vi "Main.vi"() -> ()   [LabVIEW 2020]
uses:
  Action control.ctl
  Script control.ctl
  Joystick controls.ctl
  <vilib>/Platform/TimedLoop/XDataNode/timing_clust.ctl
  <vilib>/Platform/TimedLoop/XDataNode/nitl_modes.ctl
  <vilib>/Platform/TimedLoop/XDataNode/wakeup.ctl
  8df4f0e3-bdc8-4595-ad00-b98df174246d.vi
  <vilib>/High Genius/HG_WSI_Tookit/Dependencies/Library/IMU/IMU.lvclass
  C:/Program Files (x86)/National Instruments/LabVIEW 2020/vi.lib/High Genius/HG_WSI_Tookit/Dependencies/Library/HG_LIB/HG_LIB.lvclass
  <vilib>/High Genius/HG_WSI_Tookit/Dependencies/Library/Analog In/Analog In.lvclass
  <vilib>/High Genius/HG_WSI_Tookit/Dependencies/Library/PWM/PWM.lvclass
  <vilib>/High Genius/HG_WSI_Tookit/Dependencies/Library/Digital Input and Output/Digital Input and Output.lvclass
  <vilib>/High Genius/HG_WSI_Tookit/Dependencies/Library/TitanENC/TitanENC.lvclass
  <vilib>/High Genius/HG_WSI_Tookit/Dependencies/Library/CAN/CAN.lvclass
  <vilib>/High Genius/HG_WSI_Tookit/Dependencies/Library/IIC/IIC.lvclass
  <vilib>/High Genius/HG_WSI_Tookit/Dependencies/Library/ISQ/ISQ.lvclass
  <vilib>/High Genius/HG_WSI_Tookit/Dependencies/Library/Pulse/Pulse.lvclass
  <vilib>/Platform/TimedLoop/XDataNode/XDataNode.xnode
  <vilib>/High Genius/HG_WSI_Tookit/Dependencies/Library/HG_LIB/HG_LIB.lvclass
  <vilib>/Platform/TimedLoop/XDataNode/XDNodeRunTimeDep.lvlib
panel:
  out "Waveform Chart 2":dbl(graph)=40.0
  out "Waveform Chart":dbl(graph)
  out "Volage":dbl(knob) scale=12.0..15.0
  in  "GPS Start":cluster{"X":dbl, "Y":dbl, "Angle ":i16}={"X"=166.0, "Y"=34.0, "Angle "=90}
  in  "GPS True":cluster{"X":dbl, "Y":dbl, "Z":dbl}
  in  "GPS":cluster{"X":dbl, "Y":dbl, "Angle ":i16}
  in  "Set GPS":cluster{"Set":bool, "X":dbl, "Y":dbl, "Z":dbl}
  in  "Block Rotate":bool
  in  "Tab Script":T1(tab)
  out "Array 0":T3(array[cluster])=[{"Activ"=FALSE, "X"=0.0, "Y"=0.0, "Z"=0.0, "Div"=0, "Set 1"=FALSE, "Set 2"=FALSE, "Set 3"=FALSE, "Skip"=FALSE, "action"=enum."Start"}, {"Activ"=FALSE, "X"=200.0, "Y"=113.0, "Z"=0.0, "Div"=0, "Set 1"=FALSE, "Set 2"=FALSE, "Set 3"=FALSE, "Skip"=FALSE, "action"=enum."Move"}, {"Activ"=FALSE, "X"=3.0, "Y"=0.0, "Z"=0.0, "Div"=0, "Set 1"=FALSE, "Set 2"=FALSE, "Set 3"=FALSE, "Skip"=FALSE, "action"=enum."Smooth pause"}, {"Activ"=FALSE, "X"=0.0, "Y"=0.0, "Z"=0.0, "Div"=0, "Set 1"=FALSE, "Set 2"=FALSE, "Set 3"=FALSE, "Skip"=FALSE, "action"=enum."Move"}, {"Activ"=FALSE, "X"=200.0, "Y"=50.0, "Z"=0.0, "Div"=0, "Set 1"=FALSE, "Set 2"=FALSE, "Set 3"=FALSE, "Skip"=FALSE, "action"=enum."Move"}, {"Activ"=FALSE, "X"=1.0, "Y"=0.0, "Z"=0.0, "Div"=0, "Set 1"=FALSE, "Set 2"=FALSE, "Set 3"=FALSE, "Skip"=FALSE, "action"=enum."Smooth pause"}, {"Activ"=FALSE, "X"=90.0, "Y"=0.0, "Z"=0.0, "Div"=0, "Set 1"=FALSE, "Set 2"=FALSE, "Set 3"=FALSE, "Skip"=FALSE, "action"=enum."Rotation"}, {"Activ"=FALSE, "X"=90.0, "Y"=0.0, "Z"=0.0, "Div"=0, "Set 1"=FALSE, "Set 2"=FALSE, "Set 3"=FALSE, "Skip"=FALSE, "action"=enum."Rotation"}, {"Activ"=FALSE, "X"=90.0, "Y"=0.0, "Z"=0.0, "Div"=0, "Set 1"=FALSE, "Set 2"=FALSE, "Set 3"=FALSE, "Skip"=FALSE, "action"=enum."Rotation"}, {"Activ"=FALSE, "X"=1.0, "Y"=0.0, "Z"=0.0, "Div"=0, "Set 1"=FALSE, "Set 2"=FALSE, "Set 3"=FALSE, "Skip"=FALSE, "action"=enum."Smooth pause"}, {"Activ"=FALSE, "X"=90.0, "Y"=0.0, "Z"=0.0, "Div"=0, "Set 1"=FALSE, "Set 2"=FALSE, "Set 3"=FALSE, "Skip"=FALSE, "action"=enum."Rotation Correct"}, {"Activ"=TRUE, "X"=0.0, "Y"=0.0, "Z"=0.0, "Div"=0, "Set 1"=FALSE, "Set 2"=FALSE, "Set 3"=FALSE, "Skip"=FALSE, "action"=enum."End"}]
  in  "Array 1":T3(array[cluster])=[{"Activ"=FALSE, "X"=0.0, "Y"=0.0, "Z"=0.0, "Div"=0, "Set 1"=FALSE, "Set 2"=FALSE, "Set 3"=FALSE, "Skip"=FALSE, "action"=enum."Start"}, {"Activ"=FALSE, "X"=0.0, "Y"=0.0, "Z"=0.0, "Div"=0, "Set 1"=FALSE, "Set 2"=FALSE, "Set 3"=FALSE, "Skip"=FALSE, "action"=enum."Gamepad"}, {"Activ"=FALSE, "X"=0.0, "Y"=0.0, "Z"=0.0, "Div"=0, "Set 1"=FALSE, "Set 2"=FALSE, "Set 3"=FALSE, "Skip"=FALSE, "action"=enum."Pause"}, {"Activ"=FALSE, "X"=0.0, "Y"=0.0, "Z"=0.0, "Div"=0, "Set 1"=FALSE, "Set 2"=FALSE, "Set 3"=FALSE, "Skip"=FALSE, "action"=enum."End"}]
  in  "Array 2":T3(array[cluster])=[{"Activ"=FALSE, "X"=0.0, "Y"=0.0, "Z"=0.0, "Div"=0, "Set 1"=FALSE, "Set 2"=FALSE, "Set 3"=FALSE, "Skip"=FALSE, "action"=enum."Start"}, {"Activ"=FALSE, "X"=200.0, "Y"=45.0, "Z"=0.0, "Div"=0, "Set 1"=FALSE, "Set 2"=FALSE, "Set 3"=FALSE, "Skip"=FALSE, "action"=enum."Move"}, {"Activ"=FALSE, "X"=1.0, "Y"=0.0, "Z"=0.0, "Div"=0, "Set 1"=FALSE, "Set 2"=FALSE, "Set 3"=FALSE, "Skip"=FALSE, "action"=enum."Smooth pause"}, {"Activ"=FALSE, "X"=0.0, "Y"=0.0, "Z"=0.0, "Div"=0, "Set 1"=FALSE, "Set 2"=FALSE, "Set 3"=FALSE, "Skip"=FALSE, "action"=enum."End"}]
  in  "Array 3":T3(array[cluster])=[{"Activ"=FALSE, "X"=0.0, "Y"=0.0, "Z"=0.0, "Div"=0, "Set 1"=FALSE, "Set 2"=FALSE, "Set 3"=FALSE, "Skip"=FALSE, "action"=enum."Start"}, {"Activ"=FALSE, "X"=90.0, "Y"=0.0, "Z"=0.0, "Div"=0, "Set 1"=FALSE, "Set 2"=FALSE, "Set 3"=FALSE, "Skip"=FALSE, "action"=enum."Rotation"}, {"Activ"=FALSE, "X"=90.0, "Y"=0.0, "Z"=0.0, "Div"=0, "Set 1"=FALSE, "Set 2"=FALSE, "Set 3"=FALSE, "Skip"=FALSE, "action"=enum."Rotation"}, {"Activ"=FALSE, "X"=1.0, "Y"=0.0, "Z"=0.0, "Div"=0, "Set 1"=FALSE, "Set 2"=FALSE, "Set 3"=FALSE, "Skip"=FALSE, "action"=enum."Smooth pause"}, {"Activ"=FALSE, "X"=90.0, "Y"=0.0, "Z"=0.0, "Div"=0, "Set 1"=FALSE, "Set 2"=FALSE, "Set 3"=FALSE, "Skip"=FALSE, "action"=enum."Rotation Correct"}, {"Activ"=FALSE, "X"=1.0, "Y"=0.0, "Z"=0.0, "Div"=0, "Set 1"=FALSE, "Set 2"=FALSE, "Set 3"=FALSE, "Skip"=FALSE, "action"=enum."Smooth pause"}, {"Activ"=FALSE, "X"=70.0, "Y"=0.0, "Z"=0.0, "Div"=0, "Set 1"=FALSE, "Set 2"=FALSE, "Set 3"=FALSE, "Skip"=FALSE, "action"=enum."Move"}, {"Activ"=FALSE, "X"=1.0, "Y"=0.0, "Z"=0.0, "Div"=0, "Set 1"=FALSE, "Set 2"=FALSE, "Set 3"=FALSE, "Skip"=FALSE, "action"=enum."Smooth pause"}, {"Activ"=FALSE, "X"=180.0, "Y"=0.0, "Z"=0.0, "Div"=0, "Set 1"=FALSE, "Set 2"=FALSE, "Set 3"=FALSE, "Skip"=FALSE, "action"=enum."Rotation"}, {"Activ"=FALSE, "X"=90.0, "Y"=0.0, "Z"=0.0, "Div"=0, "Set 1"=FALSE, "Set 2"=FALSE, "Set 3"=FALSE, "Skip"=FALSE, "action"=enum."Rotation"}, {"Activ"=FALSE, "X"=1.0, "Y"=0.0, "Z"=0.0, "Div"=0, "Set 1"=FALSE, "Set 2"=FALSE, "Set 3"=FALSE, "Skip"=FALSE, "action"=enum."Smooth pause"}, {"Activ"=FALSE, "X"=90.0, "Y"=0.0, "Z"=0.0, "Div"=0, "Set 1"=FALSE, "Set 2"=FALSE, "Set 3"=FALSE, "Skip"=FALSE, "action"=enum."Rotation Correct"}, {"Activ"=FALSE, "X"=1.0, "Y"=0.0, "Z"=0.0, "Div"=0, "Set 1"=FALSE, "Set 2"=FALSE, "Set 3"=FALSE, "Skip"=FALSE, "action"=enum."Smooth pause"}, {"Activ"=FALSE, "X"=240.0, "Y"=40.0, "Z"=0.0, "Div"=0, "Set 1"=FALSE, "Set 2"=FALSE, "Set 3"=FALSE, "Skip"=FALSE, "action"=enum."Move"}, {"Activ"=FALSE, "X"=1.0, "Y"=0.0, "Z"=0.0, "Div"=0, "Set 1"=FALSE, "Set 2"=FALSE, "Set 3"=FALSE, "Skip"=FALSE, "action"=enum."Smooth pause"}, {"Activ"=FALSE, "X"=-90.0, "Y"=0.0, "Z"=0.0, "Div"=0, "Set 1"=FALSE, "Set 2"=FALSE, "Set 3"=FALSE, "Skip"=FALSE, "action"=enum."Rotation"}, {"Activ"=FALSE, "X"=1.0, "Y"=0.0, "Z"=0.0, "Div"=0, "Set 1"=FALSE, "Set 2"=FALSE, "Set 3"=FALSE, "Skip"=FALSE, "action"=enum."Smooth pause"}, {"Activ"=FALSE, "X"=1.0, "Y"=0.0, "Z"=0.0, "Div"=0, "Set 1"=FALSE, "Set 2"=FALSE, "Set 3"=FALSE, "Skip"=FALSE, "action"=enum."Smooth pause"}, {"Activ"=FALSE, "X"=50.0, "Y"=0.0, "Z"=0.0, "Div"=0, "Set 1"=FALSE, "Set 2"=FALSE, "Set 3"=FALSE, "Skip"=FALSE, "action"=enum."Move"}, {"Activ"=FALSE, "X"=1.0, "Y"=0.0, "Z"=0.0, "Div"=0, "Set 1"=FALSE, "Set 2"=FALSE, "Set 3"=FALSE, "Skip"=FALSE, "action"=enum."Smooth pause"}, {"Activ"=FALSE, "X"=720.0, "Y"=0.0, "Z"=0.0, "Div"=0, "Set 1"=FALSE, "Set 2"=FALSE, "Set 3"=FALSE, "Skip"=FALSE, "action"=enum."Rotation"}, {"Activ"=FALSE, "X"=1.0, "Y"=0.0, "Z"=0.0, "Div"=0, "Set 1"=FALSE, "Set 2"=FALSE, "Set 3"=FALSE, "Skip"=FALSE, "action"=enum."Smooth pause"}, {"Activ"=FALSE, "X"=0.0, "Y"=0.0, "Z"=0.0, "Div"=0, "Set 1"=FALSE, "Set 2"=FALSE, "Set 3"=FALSE, "Skip"=FALSE, "action"=enum."End"}]
  in  "Array 4":T3(array[cluster])
  in  "Array 5":T3(array[cluster])
  in  "Array 6":T3(array[cluster])
  in  "Array 7":T3(array[cluster])
  in  "Array 8":T3(array[cluster])
  in  "Array 9":T3(array[cluster])
  in  "Array 10":T3(array[cluster])
  in  "Array 11":T3(array[cluster])
  in  "Array 12":T3(array[cluster])
  in  "Array 13":T3(array[cluster])
  in  "Array 14":T3(array[cluster])=[{"Activ"=FALSE, "X"=270.0, "Y"=0.0, "Z"=0.0, "Div"=0, "Set 1"=FALSE, "Set 2"=FALSE, "Set 3"=FALSE, "Skip"=FALSE, "action"=enum."Rotation"}, {"Activ"=FALSE, "X"=0.0, "Y"=0.0, "Z"=0.0, "Div"=0, "Set 1"=FALSE, "Set 2"=FALSE, "Set 3"=FALSE, "Skip"=FALSE, "action"=enum."Smooth pause"}, {"Activ"=FALSE, "X"=270.0, "Y"=0.0, "Z"=0.0, "Div"=0, "Set 1"=FALSE, "Set 2"=FALSE, "Set 3"=FALSE, "Skip"=FALSE, "action"=enum."Rotation Correct"}, {"Activ"=FALSE, "X"=50.0, "Y"=0.0, "Z"=0.0, "Div"=0, "Set 1"=FALSE, "Set 2"=FALSE, "Set 3"=FALSE, "Skip"=FALSE, "action"=enum."Move"}, {"Activ"=FALSE, "X"=0.0, "Y"=0.0, "Z"=0.0, "Div"=0, "Set 1"=FALSE, "Set 2"=FALSE, "Set 3"=FALSE, "Skip"=FALSE, "action"=enum."Smooth pause"}, {"Activ"=FALSE, "X"=90.0, "Y"=0.0, "Z"=0.0, "Div"=0, "Set 1"=FALSE, "Set 2"=FALSE, "Set 3"=FALSE, "Skip"=FALSE, "action"=enum."Rotation"}, {"Activ"=FALSE, "X"=0.0, "Y"=0.0, "Z"=0.0, "Div"=0, "Set 1"=FALSE, "Set 2"=FALSE, "Set 3"=FALSE, "Skip"=FALSE, "action"=enum."Pause"}, {"Activ"=FALSE, "X"=90.0, "Y"=0.0, "Z"=0.0, "Div"=0, "Set 1"=FALSE, "Set 2"=FALSE, "Set 3"=FALSE, "Skip"=FALSE, "action"=enum."Rotation Correct"}, {"Activ"=FALSE, "X"=50.0, "Y"=0.0, "Z"=0.0, "Div"=0, "Set 1"=FALSE, "Set 2"=FALSE, "Set 3"=FALSE, "Skip"=FALSE, "action"=enum."Move"}, {"Activ"=FALSE, "X"=0.0, "Y"=0.0, "Z"=0.0, "Div"=0, "Set 1"=FALSE, "Set 2"=FALSE, "Set 3"=FALSE, "Skip"=FALSE, "action"=enum."Lift"}, {"Activ"=FALSE, "X"=180.0, "Y"=0.0, "Z"=0.0, "Div"=0, "Set 1"=FALSE, "Set 2"=FALSE, "Set 3"=FALSE, "Skip"=FALSE, "action"=enum."Rotation"}, {"Activ"=FALSE, "X"=0.0, "Y"=0.0, "Z"=0.0, "Div"=0, "Set 1"=FALSE, "Set 2"=FALSE, "Set 3"=FALSE, "Skip"=FALSE, "action"=enum."Smooth pause"}, {"Activ"=FALSE, "X"=180.0, "Y"=0.0, "Z"=0.0, "Div"=0, "Set 1"=FALSE, "Set 2"=FALSE, "Set 3"=FALSE, "Skip"=FALSE, "action"=enum."Rotation Correct"}, {"Activ"=FALSE, "X"=100.0, "Y"=0.0, "Z"=0.0, "Div"=0, "Set 1"=FALSE, "Set 2"=FALSE, "Set 3"=FALSE, "Skip"=FALSE, "action"=enum."Move"}, {"Activ"=FALSE, "X"=0.0, "Y"=0.0, "Z"=0.0, "Div"=0, "Set 1"=FALSE, "Set 2"=FALSE, "Set 3"=FALSE, "Skip"=FALSE, "action"=enum."Smooth pause"}, {"Activ"=FALSE, "X"=90.0, "Y"=0.0, "Z"=0.0, "Div"=0, "Set 1"=FALSE, "Set 2"=FALSE, "Set 3"=FALSE, "Skip"=FALSE, "action"=enum."Rotation"}, {"Activ"=FALSE, "X"=0.0, "Y"=0.0, "Z"=0.0, "Div"=0, "Set 1"=FALSE, "Set 2"=FALSE, "Set 3"=FALSE, "Skip"=FALSE, "action"=enum."Smooth pause"}, {"Activ"=FALSE, "X"=90.0, "Y"=0.0, "Z"=0.0, "Div"=0, "Set 1"=FALSE, "Set 2"=FALSE, "Set 3"=FALSE, "Skip"=FALSE, "action"=enum."Rotation Correct"}, {"Activ"=FALSE, "X"=8000.0, "Y"=45.0, "Z"=0.0, "Div"=0, "Set 1"=FALSE, "Set 2"=FALSE, "Set 3"=FALSE, "Skip"=FALSE, "action"=enum."Move"}]
  in  "Array 15":T3(array[cluster])=[{"Activ"=FALSE, "X"=90.0, "Y"=0.0, "Z"=0.0, "Div"=0, "Set 1"=FALSE, "Set 2"=FALSE, "Set 3"=FALSE, "Skip"=FALSE, "action"=enum."Rotation"}, {"Activ"=FALSE, "X"=1.0, "Y"=0.0, "Z"=0.0, "Div"=0, "Set 1"=FALSE, "Set 2"=FALSE, "Set 3"=FALSE, "Skip"=FALSE, "action"=enum."Smooth pause"}, {"Activ"=FALSE, "X"=90.0, "Y"=0.0, "Z"=0.0, "Div"=0, "Set 1"=FALSE, "Set 2"=FALSE, "Set 3"=FALSE, "Skip"=FALSE, "action"=enum."Rotation Correct"}, {"Activ"=FALSE, "X"=50.0, "Y"=0.0, "Z"=0.0, "Div"=0, "Set 1"=FALSE, "Set 2"=FALSE, "Set 3"=FALSE, "Skip"=FALSE, "action"=enum."Move"}, {"Activ"=FALSE, "X"=1.0, "Y"=0.0, "Z"=0.0, "Div"=0, "Set 1"=FALSE, "Set 2"=FALSE, "Set 3"=FALSE, "Skip"=FALSE, "action"=enum."Smooth pause"}, {"Activ"=FALSE, "X"=270.0, "Y"=0.0, "Z"=0.0, "Div"=0, "Set 1"=FALSE, "Set 2"=FALSE, "Set 3"=FALSE, "Skip"=FALSE, "action"=enum."Rotation"}, {"Activ"=FALSE, "X"=1.0, "Y"=0.0, "Z"=0.0, "Div"=0, "Set 1"=FALSE, "Set 2"=FALSE, "Set 3"=FALSE, "Skip"=FALSE, "action"=enum."Smooth pause"}, {"Activ"=FALSE, "X"=270.0, "Y"=0.0, "Z"=0.0, "Div"=0, "Set 1"=FALSE, "Set 2"=FALSE, "Set 3"=FALSE, "Skip"=FALSE, "action"=enum."Rotation Correct"}, {"Activ"=FALSE, "X"=50.0, "Y"=0.0, "Z"=0.0, "Div"=0, "Set 1"=FALSE, "Set 2"=FALSE, "Set 3"=FALSE, "Skip"=FALSE, "action"=enum."Move"}, {"Activ"=FALSE, "X"=0.0, "Y"=0.0, "Z"=0.0, "Div"=0, "Set 1"=FALSE, "Set 2"=FALSE, "Set 3"=FALSE, "Skip"=FALSE, "action"=enum."Lift"}, {"Activ"=FALSE, "X"=180.0, "Y"=0.0, "Z"=0.0, "Div"=0, "Set 1"=FALSE, "Set 2"=FALSE, "Set 3"=FALSE, "Skip"=FALSE, "action"=enum."Rotation"}, {"Activ"=FALSE, "X"=1.0, "Y"=0.0, "Z"=0.0, "Div"=0, "Set 1"=FALSE, "Set 2"=FALSE, "Set 3"=FALSE, "Skip"=FALSE, "action"=enum."Smooth pause"}, {"Activ"=FALSE, "X"=180.0, "Y"=0.0, "Z"=0.0, "Div"=0, "Set 1"=FALSE, "Set 2"=FALSE, "Set 3"=FALSE, "Skip"=FALSE, "action"=enum."Rotation Correct"}, {"Activ"=FALSE, "X"=100.0, "Y"=0.0, "Z"=0.0, "Div"=0, "Set 1"=FALSE, "Set 2"=FALSE, "Set 3"=FALSE, "Skip"=FALSE, "action"=enum."Move"}, {"Activ"=FALSE, "X"=0.0, "Y"=0.0, "Z"=0.0, "Div"=0, "Set 1"=FALSE, "Set 2"=FALSE, "Set 3"=FALSE, "Skip"=FALSE, "action"=enum."Smooth pause"}, {"Activ"=FALSE, "X"=270.0, "Y"=0.0, "Z"=0.0, "Div"=0, "Set 1"=FALSE, "Set 2"=FALSE, "Set 3"=FALSE, "Skip"=FALSE, "action"=enum."Rotation"}, {"Activ"=FALSE, "X"=1.0, "Y"=0.0, "Z"=0.0, "Div"=0, "Set 1"=FALSE, "Set 2"=FALSE, "Set 3"=FALSE, "Skip"=FALSE, "action"=enum."Smooth pause"}, {"Activ"=FALSE, "X"=270.0, "Y"=0.0, "Z"=0.0, "Div"=0, "Set 1"=FALSE, "Set 2"=FALSE, "Set 3"=FALSE, "Skip"=FALSE, "action"=enum."Rotation Correct"}, {"Activ"=FALSE, "X"=8000.0, "Y"=45.0, "Z"=0.0, "Div"=0, "Set 1"=FALSE, "Set 2"=FALSE, "Set 3"=FALSE, "Skip"=FALSE, "action"=enum."Move"}]
  in  "Array 16":T3(array[cluster])=[{"Activ"=FALSE, "X"=270.0, "Y"=0.0, "Z"=0.0, "Div"=0, "Set 1"=FALSE, "Set 2"=FALSE, "Set 3"=FALSE, "Skip"=FALSE, "action"=enum."Rotation"}, {"Activ"=FALSE, "X"=1.0, "Y"=0.0, "Z"=0.0, "Div"=0, "Set 1"=FALSE, "Set 2"=FALSE, "Set 3"=FALSE, "Skip"=FALSE, "action"=enum."Smooth pause"}, {"Activ"=FALSE, "X"=270.0, "Y"=0.0, "Z"=0.0, "Div"=0, "Set 1"=FALSE, "Set 2"=FALSE, "Set 3"=FALSE, "Skip"=FALSE, "action"=enum."Rotation Correct"}, {"Activ"=FALSE, "X"=50.0, "Y"=0.0, "Z"=0.0, "Div"=0, "Set 1"=FALSE, "Set 2"=FALSE, "Set 3"=FALSE, "Skip"=FALSE, "action"=enum."Move"}, {"Activ"=FALSE, "X"=1.0, "Y"=0.0, "Z"=0.0, "Div"=0, "Set 1"=FALSE, "Set 2"=FALSE, "Set 3"=FALSE, "Skip"=FALSE, "action"=enum."Smooth pause"}, {"Activ"=FALSE, "X"=90.0, "Y"=0.0, "Z"=0.0, "Div"=0, "Set 1"=FALSE, "Set 2"=FALSE, "Set 3"=FALSE, "Skip"=FALSE, "action"=enum."Rotation"}, {"Activ"=FALSE, "X"=1.0, "Y"=0.0, "Z"=0.0, "Div"=0, "Set 1"=FALSE, "Set 2"=FALSE, "Set 3"=FALSE, "Skip"=FALSE, "action"=enum."Smooth pause"}, {"Activ"=FALSE, "X"=90.0, "Y"=0.0, "Z"=0.0, "Div"=0, "Set 1"=FALSE, "Set 2"=FALSE, "Set 3"=FALSE, "Skip"=FALSE, "action"=enum."Rotation Correct"}, {"Activ"=FALSE, "X"=50.0, "Y"=0.0, "Z"=0.0, "Div"=0, "Set 1"=FALSE, "Set 2"=FALSE, "Set 3"=FALSE, "Skip"=FALSE, "action"=enum."Move"}, {"Activ"=FALSE, "X"=0.0, "Y"=0.0, "Z"=0.0, "Div"=0, "Set 1"=FALSE, "Set 2"=FALSE, "Set 3"=FALSE, "Skip"=FALSE, "action"=enum."Lift"}, {"Activ"=FALSE, "X"=180.0, "Y"=0.0, "Z"=0.0, "Div"=0, "Set 1"=FALSE, "Set 2"=FALSE, "Set 3"=FALSE, "Skip"=FALSE, "action"=enum."Rotation"}, {"Activ"=FALSE, "X"=1.0, "Y"=0.0, "Z"=0.0, "Div"=0, "Set 1"=FALSE, "Set 2"=FALSE, "Set 3"=FALSE, "Skip"=FALSE, "action"=enum."Smooth pause"}, {"Activ"=FALSE, "X"=180.0, "Y"=0.0, "Z"=0.0, "Div"=0, "Set 1"=FALSE, "Set 2"=FALSE, "Set 3"=FALSE, "Skip"=FALSE, "action"=enum."Rotation Correct"}, {"Activ"=FALSE, "X"=100.0, "Y"=0.0, "Z"=0.0, "Div"=0, "Set 1"=FALSE, "Set 2"=FALSE, "Set 3"=FALSE, "Skip"=FALSE, "action"=enum."Move"}, {"Activ"=FALSE, "X"=1.0, "Y"=0.0, "Z"=0.0, "Div"=0, "Set 1"=FALSE, "Set 2"=FALSE, "Set 3"=FALSE, "Skip"=FALSE, "action"=enum."Smooth pause"}, {"Activ"=FALSE, "X"=270.0, "Y"=0.0, "Z"=0.0, "Div"=0, "Set 1"=FALSE, "Set 2"=FALSE, "Set 3"=FALSE, "Skip"=FALSE, "action"=enum."Rotation"}, {"Activ"=FALSE, "X"=1.0, "Y"=0.0, "Z"=0.0, "Div"=0, "Set 1"=FALSE, "Set 2"=FALSE, "Set 3"=FALSE, "Skip"=FALSE, "action"=enum."Smooth pause"}, {"Activ"=FALSE, "X"=270.0, "Y"=0.0, "Z"=0.0, "Div"=0, "Set 1"=FALSE, "Set 2"=FALSE, "Set 3"=FALSE, "Skip"=FALSE, "action"=enum."Rotation Correct"}, {"Activ"=FALSE, "X"=8000.0, "Y"=45.0, "Z"=0.0, "Div"=0, "Set 1"=FALSE, "Set 2"=FALSE, "Set 3"=FALSE, "Skip"=FALSE, "action"=enum."Move"}, {"Activ"=FALSE, "X"=1.0, "Y"=0.0, "Z"=0.0, "Div"=0, "Set 1"=FALSE, "Set 2"=FALSE, "Set 3"=FALSE, "Skip"=FALSE, "action"=enum."Smooth pause"}]
  in  "Array 17":T3(array[cluster])
  in  "Array 18":T3(array[cluster])
  in  "Array 19":T3(array[cluster])
  in  "Array 20":T3(array[cluster])=[{"Activ"=FALSE, "X"=125.0, "Y"=0.0, "Z"=0.0, "Div"=0, "Set 1"=FALSE, "Set 2"=FALSE, "Set 3"=FALSE, "Skip"=FALSE, "action"=enum."Move"}, {"Activ"=FALSE, "X"=1.0, "Y"=0.0, "Z"=0.0, "Div"=0, "Set 1"=FALSE, "Set 2"=FALSE, "Set 3"=FALSE, "Skip"=FALSE, "action"=enum."Pause"}, {"Activ"=FALSE, "X"=90.0, "Y"=0.0, "Z"=0.0, "Div"=0, "Set 1"=FALSE, "Set 2"=FALSE, "Set 3"=FALSE, "Skip"=FALSE, "action"=enum."Rotation"}, {"Activ"=FALSE, "X"=1.0, "Y"=0.0, "Z"=0.0, "Div"=0, "Set 1"=FALSE, "Set 2"=FALSE, "Set 3"=FALSE, "Skip"=FALSE, "action"=enum."Smooth pause"}, {"Activ"=FALSE, "X"=90.0, "Y"=0.0, "Z"=0.0, "Div"=0, "Set 1"=FALSE, "Set 2"=FALSE, "Set 3"=FALSE, "Skip"=FALSE, "action"=enum."Rotation Correct"}, {"Activ"=FALSE, "X"=0.0, "Y"=0.0, "Z"=0.0, "Div"=0, "Set 1"=FALSE, "Set 2"=FALSE, "Set 3"=FALSE, "Skip"=FALSE, "action"=enum."Move"}, {"Activ"=FALSE, "X"=210.0, "Y"=0.0, "Z"=0.0, "Div"=0, "Set 1"=FALSE, "Set 2"=FALSE, "Set 3"=FALSE, "Skip"=FALSE, "action"=enum."Move"}, {"Activ"=FALSE, "X"=1.0, "Y"=0.0, "Z"=0.0, "Div"=0, "Set 1"=FALSE, "Set 2"=FALSE, "Set 3"=FALSE, "Skip"=FALSE, "action"=enum."Pause"}, {"Activ"=FALSE, "X"=90.0, "Y"=0.0, "Z"=0.0, "Div"=0, "Set 1"=FALSE, "Set 2"=FALSE, "Set 3"=FALSE, "Skip"=FALSE, "action"=enum."Rotation"}, {"Activ"=FALSE, "X"=90.0, "Y"=0.0, "Z"=0.0, "Div"=0, "Set 1"=FALSE, "Set 2"=FALSE, "Set 3"=FALSE, "Skip"=FALSE, "action"=enum."Rotation"}, {"Activ"=FALSE, "X"=90.0, "Y"=0.0, "Z"=0.0, "Div"=0, "Set 1"=FALSE, "Set 2"=FALSE, "Set 3"=FALSE, "Skip"=FALSE, "action"=enum."Rotation"}, {"Activ"=FALSE, "X"=1.0, "Y"=0.0, "Z"=0.0, "Div"=0, "Set 1"=FALSE, "Set 2"=FALSE, "Set 3"=FALSE, "Skip"=FALSE, "action"=enum."Smooth pause"}, {"Activ"=FALSE, "X"=90.0, "Y"=0.0, "Z"=0.0, "Div"=0, "Set 1"=FALSE, "Set 2"=FALSE, "Set 3"=FALSE, "Skip"=FALSE, "action"=enum."Rotation Correct"}, {"Activ"=FALSE, "X"=0.0, "Y"=0.0, "Z"=0.0, "Div"=0, "Set 1"=FALSE, "Set 2"=FALSE, "Set 3"=FALSE, "Skip"=FALSE, "action"=enum."Move"}, {"Activ"=FALSE, "X"=135.0, "Y"=0.0, "Z"=0.0, "Div"=0, "Set 1"=FALSE, "Set 2"=FALSE, "Set 3"=FALSE, "Skip"=FALSE, "action"=enum."Move"}, {"Activ"=FALSE, "X"=1.0, "Y"=0.0, "Z"=0.0, "Div"=0, "Set 1"=FALSE, "Set 2"=FALSE, "Set 3"=FALSE, "Skip"=FALSE, "action"=enum."Smooth pause"}, {"Activ"=FALSE, "X"=90.0, "Y"=0.0, "Z"=0.0, "Div"=0, "Set 1"=FALSE, "Set 2"=FALSE, "Set 3"=FALSE, "Skip"=FALSE, "action"=enum."Rotation"}, {"Activ"=FALSE, "X"=1.0, "Y"=0.0, "Z"=0.0, "Div"=0, "Set 1"=FALSE, "Set 2"=FALSE, "Set 3"=FALSE, "Skip"=FALSE, "action"=enum."Smooth pause"}, {"Activ"=FALSE, "X"=0.0, "Y"=0.0, "Z"=0.0, "Div"=0, "Set 1"=FALSE, "Set 2"=FALSE, "Set 3"=FALSE, "Skip"=FALSE, "action"=enum."Move"}, {"Activ"=FALSE, "X"=200.0, "Y"=100.0, "Z"=0.0, "Div"=0, "Set 1"=FALSE, "Set 2"=FALSE, "Set 3"=FALSE, "Skip"=FALSE, "action"=enum."Move"}, {"Activ"=FALSE, "X"=0.0, "Y"=0.0, "Z"=0.0, "Div"=0, "Set 1"=TRUE, "Set 2"=FALSE, "Set 3"=FALSE, "Skip"=FALSE, "action"=enum."Camera"}]
  in  "Array 21":T3(array[cluster])=[{"Activ"=FALSE, "X"=0.0, "Y"=0.0, "Z"=0.0, "Div"=0, "Set 1"=FALSE, "Set 2"=FALSE, "Set 3"=FALSE, "Skip"=FALSE, "action"=enum."Start"}, {"Activ"=FALSE, "X"=180.0, "Y"=0.0, "Z"=0.0, "Div"=0, "Set 1"=FALSE, "Set 2"=FALSE, "Set 3"=FALSE, "Skip"=FALSE, "action"=enum."Rotation"}, {"Activ"=FALSE, "X"=90.0, "Y"=0.0, "Z"=0.0, "Div"=0, "Set 1"=FALSE, "Set 2"=FALSE, "Set 3"=FALSE, "Skip"=FALSE, "action"=enum."Rotation"}, {"Activ"=FALSE, "X"=1.0, "Y"=0.0, "Z"=0.0, "Div"=0, "Set 1"=FALSE, "Set 2"=FALSE, "Set 3"=FALSE, "Skip"=FALSE, "action"=enum."Smooth pause"}, {"Activ"=FALSE, "X"=90.0, "Y"=0.0, "Z"=0.0, "Div"=0, "Set 1"=FALSE, "Set 2"=FALSE, "Set 3"=FALSE, "Skip"=FALSE, "action"=enum."Rotation Correct"}, {"Activ"=FALSE, "X"=1.0, "Y"=0.0, "Z"=0.0, "Div"=0, "Set 1"=FALSE, "Set 2"=FALSE, "Set 3"=FALSE, "Skip"=FALSE, "action"=enum."Smooth pause"}, {"Activ"=FALSE, "X"=30.0, "Y"=0.0, "Z"=0.0, "Div"=0, "Set 1"=FALSE, "Set 2"=FALSE, "Set 3"=FALSE, "Skip"=FALSE, "action"=enum."Move"}, {"Activ"=FALSE, "X"=1.0, "Y"=0.0, "Z"=0.0, "Div"=0, "Set 1"=FALSE, "Set 2"=FALSE, "Set 3"=FALSE, "Skip"=FALSE, "action"=enum."Smooth pause"}, {"Activ"=FALSE, "X"=180.0, "Y"=0.0, "Z"=0.0, "Div"=0, "Set 1"=FALSE, "Set 2"=FALSE, "Set 3"=FALSE, "Skip"=FALSE, "action"=enum."Rotation"}, {"Activ"=FALSE, "X"=90.0, "Y"=0.0, "Z"=0.0, "Div"=0, "Set 1"=FALSE, "Set 2"=FALSE, "Set 3"=FALSE, "Skip"=FALSE, "action"=enum."Rotation"}, {"Activ"=FALSE, "X"=1.0, "Y"=0.0, "Z"=0.0, "Div"=0, "Set 1"=FALSE, "Set 2"=FALSE, "Set 3"=FALSE, "Skip"=FALSE, "action"=enum."Smooth pause"}, {"Activ"=FALSE, "X"=90.0, "Y"=0.0, "Z"=0.0, "Div"=0, "Set 1"=FALSE, "Set 2"=FALSE, "Set 3"=FALSE, "Skip"=FALSE, "action"=enum."Rotation Correct"}, {"Activ"=FALSE, "X"=1.0, "Y"=0.0, "Z"=0.0, "Div"=0, "Set 1"=FALSE, "Set 2"=FALSE, "Set 3"=FALSE, "Skip"=FALSE, "action"=enum."Smooth pause"}, {"Activ"=FALSE, "X"=500.0, "Y"=50.0, "Z"=0.0, "Div"=0, "Set 1"=FALSE, "Set 2"=FALSE, "Set 3"=FALSE, "Skip"=FALSE, "action"=enum."Move"}, {"Activ"=FALSE, "X"=1.0, "Y"=0.0, "Z"=0.0, "Div"=0, "Set 1"=FALSE, "Set 2"=FALSE, "Set 3"=FALSE, "Skip"=FALSE, "action"=enum."Smooth pause"}]
  in  "Array 22":T3(array[cluster])=[{"Activ"=FALSE, "X"=180.0, "Y"=0.0, "Z"=0.0, "Div"=0, "Set 1"=FALSE, "Set 2"=FALSE, "Set 3"=FALSE, "Skip"=FALSE, "action"=enum."Rotation"}, {"Activ"=FALSE, "X"=90.0, "Y"=0.0, "Z"=0.0, "Div"=0, "Set 1"=FALSE, "Set 2"=FALSE, "Set 3"=FALSE, "Skip"=FALSE, "action"=enum."Rotation"}, {"Activ"=FALSE, "X"=1.0, "Y"=0.0, "Z"=0.0, "Div"=0, "Set 1"=FALSE, "Set 2"=FALSE, "Set 3"=FALSE, "Skip"=FALSE, "action"=enum."Smooth pause"}, {"Activ"=FALSE, "X"=90.0, "Y"=0.0, "Z"=0.0, "Div"=0, "Set 1"=FALSE, "Set 2"=FALSE, "Set 3"=FALSE, "Skip"=FALSE, "action"=enum."Rotation Correct"}, {"Activ"=FALSE, "X"=0.0, "Y"=0.0, "Z"=0.0, "Div"=0, "Set 1"=FALSE, "Set 2"=FALSE, "Set 3"=FALSE, "Skip"=FALSE, "action"=enum."Move"}, {"Activ"=FALSE, "X"=330.0, "Y"=0.0, "Z"=0.0, "Div"=0, "Set 1"=FALSE, "Set 2"=FALSE, "Set 3"=FALSE, "Skip"=FALSE, "action"=enum."Move"}, {"Activ"=FALSE, "X"=1.0, "Y"=0.0, "Z"=0.0, "Div"=0, "Set 1"=FALSE, "Set 2"=FALSE, "Set 3"=FALSE, "Skip"=FALSE, "action"=enum."Smooth pause"}, {"Activ"=FALSE, "X"=180.0, "Y"=0.0, "Z"=0.0, "Div"=0, "Set 1"=FALSE, "Set 2"=FALSE, "Set 3"=FALSE, "Skip"=FALSE, "action"=enum."Rotation"}, {"Activ"=FALSE, "X"=90.0, "Y"=0.0, "Z"=0.0, "Div"=0, "Set 1"=FALSE, "Set 2"=FALSE, "Set 3"=FALSE, "Skip"=FALSE, "action"=enum."Rotation"}, {"Activ"=FALSE, "X"=1.0, "Y"=0.0, "Z"=0.0, "Div"=0, "Set 1"=FALSE, "Set 2"=FALSE, "Set 3"=FALSE, "Skip"=FALSE, "action"=enum."Smooth pause"}, {"Activ"=FALSE, "X"=90.0, "Y"=0.0, "Z"=0.0, "Div"=0, "Set 1"=FALSE, "Set 2"=FALSE, "Set 3"=FALSE, "Skip"=FALSE, "action"=enum."Rotation Correct"}, {"Activ"=FALSE, "X"=0.0, "Y"=0.0, "Z"=0.0, "Div"=0, "Set 1"=FALSE, "Set 2"=FALSE, "Set 3"=FALSE, "Skip"=FALSE, "action"=enum."Move"}, {"Activ"=FALSE, "X"=100.0, "Y"=0.0, "Z"=0.0, "Div"=0, "Set 1"=FALSE, "Set 2"=FALSE, "Set 3"=FALSE, "Skip"=FALSE, "action"=enum."Move"}]
  in  "Array 23":T3(array[cluster])=[{"Activ"=FALSE, "X"=0.0, "Y"=0.0, "Z"=0.0, "Div"=0, "Set 1"=FALSE, "Set 2"=FALSE, "Set 3"=FALSE, "Skip"=FALSE, "action"=enum."Move"}, {"Activ"=FALSE, "X"=90.0, "Y"=0.0, "Z"=0.0, "Div"=0, "Set 1"=FALSE, "Set 2"=FALSE, "Set 3"=FALSE, "Skip"=FALSE, "action"=enum."Rotation"}, {"Activ"=FALSE, "X"=90.0, "Y"=0.0, "Z"=0.0, "Div"=0, "Set 1"=FALSE, "Set 2"=FALSE, "Set 3"=FALSE, "Skip"=FALSE, "action"=enum."Rotation"}, {"Activ"=FALSE, "X"=90.0, "Y"=0.0, "Z"=0.0, "Div"=0, "Set 1"=FALSE, "Set 2"=FALSE, "Set 3"=FALSE, "Skip"=FALSE, "action"=enum."Rotation"}, {"Activ"=FALSE, "X"=1.0, "Y"=0.0, "Z"=0.0, "Div"=0, "Set 1"=FALSE, "Set 2"=FALSE, "Set 3"=FALSE, "Skip"=FALSE, "action"=enum."Smooth pause"}, {"Activ"=FALSE, "X"=90.0, "Y"=0.0, "Z"=0.0, "Div"=0, "Set 1"=FALSE, "Set 2"=FALSE, "Set 3"=FALSE, "Skip"=FALSE, "action"=enum."Rotation Correct"}, {"Activ"=FALSE, "X"=0.0, "Y"=0.0, "Z"=0.0, "Div"=0, "Set 1"=FALSE, "Set 2"=FALSE, "Set 3"=FALSE, "Skip"=FALSE, "action"=enum."Move"}, {"Activ"=FALSE, "X"=700.0, "Y"=75.0, "Z"=0.0, "Div"=0, "Set 1"=FALSE, "Set 2"=FALSE, "Set 3"=FALSE, "Skip"=FALSE, "action"=enum."Move"}, {"Activ"=FALSE, "X"=1.0, "Y"=0.0, "Z"=0.0, "Div"=0, "Set 1"=FALSE, "Set 2"=FALSE, "Set 3"=FALSE, "Skip"=FALSE, "action"=enum."Smooth pause"}, {"Activ"=FALSE, "X"=90.0, "Y"=0.0, "Z"=0.0, "Div"=0, "Set 1"=FALSE, "Set 2"=FALSE, "Set 3"=FALSE, "Skip"=FALSE, "action"=enum."Rotation"}, {"Activ"=FALSE, "X"=90.0, "Y"=0.0, "Z"=0.0, "Div"=0, "Set 1"=FALSE, "Set 2"=FALSE, "Set 3"=FALSE, "Skip"=FALSE, "action"=enum."Rotation"}, {"Activ"=FALSE, "X"=90.0, "Y"=0.0, "Z"=0.0, "Div"=0, "Set 1"=FALSE, "Set 2"=FALSE, "Set 3"=FALSE, "Skip"=FALSE, "action"=enum."Rotation"}, {"Activ"=FALSE, "X"=1.0, "Y"=0.0, "Z"=0.0, "Div"=0, "Set 1"=FALSE, "Set 2"=FALSE, "Set 3"=FALSE, "Skip"=FALSE, "action"=enum."Smooth pause"}, {"Activ"=FALSE, "X"=90.0, "Y"=0.0, "Z"=0.0, "Div"=0, "Set 1"=FALSE, "Set 2"=FALSE, "Set 3"=FALSE, "Skip"=FALSE, "action"=enum."Rotation Correct"}, {"Activ"=FALSE, "X"=0.0, "Y"=0.0, "Z"=0.0, "Div"=0, "Set 1"=FALSE, "Set 2"=FALSE, "Set 3"=FALSE, "Skip"=FALSE, "action"=enum."Move"}, {"Activ"=FALSE, "X"=200.0, "Y"=50.0, "Z"=0.0, "Div"=0, "Set 1"=FALSE, "Set 2"=FALSE, "Set 3"=FALSE, "Skip"=FALSE, "action"=enum."Move"}, {"Activ"=FALSE, "X"=1.0, "Y"=0.0, "Z"=0.0, "Div"=0, "Set 1"=FALSE, "Set 2"=FALSE, "Set 3"=FALSE, "Skip"=FALSE, "action"=enum."Smooth pause"}]
  in  "Array 24":T3(array[cluster])=[{"Activ"=FALSE, "X"=0.0, "Y"=0.0, "Z"=0.0, "Div"=0, "Set 1"=FALSE, "Set 2"=FALSE, "Set 3"=FALSE, "Skip"=FALSE, "action"=enum."Move"}, {"Activ"=FALSE, "X"=90.0, "Y"=0.0, "Z"=0.0, "Div"=0, "Set 1"=FALSE, "Set 2"=FALSE, "Set 3"=FALSE, "Skip"=FALSE, "action"=enum."Rotation"}, {"Activ"=FALSE, "X"=90.0, "Y"=0.0, "Z"=0.0, "Div"=0, "Set 1"=FALSE, "Set 2"=FALSE, "Set 3"=FALSE, "Skip"=FALSE, "action"=enum."Rotation"}, {"Activ"=FALSE, "X"=90.0, "Y"=0.0, "Z"=0.0, "Div"=0, "Set 1"=FALSE, "Set 2"=FALSE, "Set 3"=FALSE, "Skip"=FALSE, "action"=enum."Rotation"}, {"Activ"=FALSE, "X"=1.0, "Y"=0.0, "Z"=0.0, "Div"=0, "Set 1"=FALSE, "Set 2"=FALSE, "Set 3"=FALSE, "Skip"=FALSE, "action"=enum."Smooth pause"}, {"Activ"=FALSE, "X"=90.0, "Y"=0.0, "Z"=0.0, "Div"=0, "Set 1"=FALSE, "Set 2"=FALSE, "Set 3"=FALSE, "Skip"=FALSE, "action"=enum."Rotation Correct"}, {"Activ"=FALSE, "X"=0.0, "Y"=0.0, "Z"=0.0, "Div"=0, "Set 1"=FALSE, "Set 2"=FALSE, "Set 3"=FALSE, "Skip"=FALSE, "action"=enum."Move"}, {"Activ"=FALSE, "X"=680.0, "Y"=0.0, "Z"=0.0, "Div"=0, "Set 1"=FALSE, "Set 2"=FALSE, "Set 3"=FALSE, "Skip"=FALSE, "action"=enum."Move"}, {"Activ"=FALSE, "X"=1.0, "Y"=0.0, "Z"=0.0, "Div"=0, "Set 1"=FALSE, "Set 2"=FALSE, "Set 3"=FALSE, "Skip"=FALSE, "action"=enum."Smooth pause"}, {"Activ"=FALSE, "X"=90.0, "Y"=0.0, "Z"=0.0, "Div"=0, "Set 1"=FALSE, "Set 2"=FALSE, "Set 3"=FALSE, "Skip"=FALSE, "action"=enum."Rotation"}, {"Activ"=FALSE, "X"=1.0, "Y"=0.0, "Z"=0.0, "Div"=0, "Set 1"=FALSE, "Set 2"=FALSE, "Set 3"=FALSE, "Skip"=FALSE, "action"=enum."Smooth pause"}, {"Activ"=FALSE, "X"=90.0, "Y"=0.0, "Z"=0.0, "Div"=0, "Set 1"=FALSE, "Set 2"=FALSE, "Set 3"=FALSE, "Skip"=FALSE, "action"=enum."Rotation Correct"}, {"Activ"=FALSE, "X"=0.0, "Y"=0.0, "Z"=0.0, "Div"=0, "Set 1"=FALSE, "Set 2"=FALSE, "Set 3"=FALSE, "Skip"=FALSE, "action"=enum."Move"}, {"Activ"=FALSE, "X"=200.0, "Y"=50.0, "Z"=0.0, "Div"=0, "Set 1"=FALSE, "Set 2"=FALSE, "Set 3"=FALSE, "Skip"=FALSE, "action"=enum."Move"}, {"Activ"=FALSE, "X"=0.0, "Y"=0.0, "Z"=0.0, "Div"=0, "Set 1"=FALSE, "Set 2"=FALSE, "Set 3"=FALSE, "Skip"=FALSE, "action"=enum."Smooth pause"}]
  in  "Array 25":T3(array[cluster])=[{"Activ"=FALSE, "X"=180.0, "Y"=0.0, "Z"=0.0, "Div"=0, "Set 1"=FALSE, "Set 2"=FALSE, "Set 3"=FALSE, "Skip"=FALSE, "action"=enum."Rotation"}, {"Activ"=FALSE, "X"=90.0, "Y"=0.0, "Z"=0.0, "Div"=0, "Set 1"=FALSE, "Set 2"=FALSE, "Set 3"=FALSE, "Skip"=FALSE, "action"=enum."Rotation"}, {"Activ"=FALSE, "X"=1.0, "Y"=0.0, "Z"=0.0, "Div"=0, "Set 1"=FALSE, "Set 2"=FALSE, "Set 3"=FALSE, "Skip"=FALSE, "action"=enum."Smooth pause"}, {"Activ"=FALSE, "X"=90.0, "Y"=0.0, "Z"=0.0, "Div"=0, "Set 1"=FALSE, "Set 2"=FALSE, "Set 3"=FALSE, "Skip"=FALSE, "action"=enum."Rotation Correct"}, {"Activ"=FALSE, "X"=0.0, "Y"=0.0, "Z"=0.0, "Div"=0, "Set 1"=FALSE, "Set 2"=FALSE, "Set 3"=FALSE, "Skip"=FALSE, "action"=enum."Move"}, {"Activ"=FALSE, "X"=330.0, "Y"=0.0, "Z"=0.0, "Div"=0, "Set 1"=FALSE, "Set 2"=FALSE, "Set 3"=FALSE, "Skip"=FALSE, "action"=enum."Move"}, {"Activ"=FALSE, "X"=0.0, "Y"=0.0, "Z"=0.0, "Div"=0, "Set 1"=FALSE, "Set 2"=FALSE, "Set 3"=FALSE, "Skip"=FALSE, "action"=enum."Smooth pause"}, {"Activ"=FALSE, "X"=90.0, "Y"=0.0, "Z"=0.0, "Div"=0, "Set 1"=FALSE, "Set 2"=FALSE, "Set 3"=FALSE, "Skip"=FALSE, "action"=enum."Rotation"}, {"Activ"=FALSE, "X"=1.0, "Y"=0.0, "Z"=0.0, "Div"=0, "Set 1"=FALSE, "Set 2"=FALSE, "Set 3"=FALSE, "Skip"=FALSE, "action"=enum."Smooth pause"}, {"Activ"=FALSE, "X"=90.0, "Y"=0.0, "Z"=0.0, "Div"=0, "Set 1"=FALSE, "Set 2"=FALSE, "Set 3"=FALSE, "Skip"=FALSE, "action"=enum."Rotation Correct"}, {"Activ"=FALSE, "X"=0.0, "Y"=0.0, "Z"=0.0, "Div"=0, "Set 1"=FALSE, "Set 2"=FALSE, "Set 3"=FALSE, "Skip"=FALSE, "action"=enum."Move"}, {"Activ"=FALSE, "X"=100.0, "Y"=80.0, "Z"=0.0, "Div"=0, "Set 1"=FALSE, "Set 2"=FALSE, "Set 3"=FALSE, "Skip"=FALSE, "action"=enum."Move"}, {"Activ"=FALSE, "X"=1.0, "Y"=0.0, "Z"=0.0, "Div"=0, "Set 1"=FALSE, "Set 2"=FALSE, "Set 3"=FALSE, "Skip"=FALSE, "action"=enum."Smooth pause"}]
  in  "Array 26":T3(array[cluster])=[{"Activ"=FALSE, "X"=0.0, "Y"=0.0, "Z"=0.0, "Div"=0, "Set 1"=FALSE, "Set 2"=FALSE, "Set 3"=FALSE, "Skip"=FALSE, "action"=enum."Move"}, {"Activ"=FALSE, "X"=200.0, "Y"=50.0, "Z"=0.0, "Div"=0, "Set 1"=FALSE, "Set 2"=FALSE, "Set 3"=FALSE, "Skip"=FALSE, "action"=enum."Move"}, {"Activ"=FALSE, "X"=1.0, "Y"=0.0, "Z"=0.0, "Div"=0, "Set 1"=FALSE, "Set 2"=FALSE, "Set 3"=FALSE, "Skip"=FALSE, "action"=enum."Smooth pause"}, {"Activ"=FALSE, "X"=90.0, "Y"=0.0, "Z"=0.0, "Div"=0, "Set 1"=FALSE, "Set 2"=FALSE, "Set 3"=FALSE, "Skip"=FALSE, "action"=enum."Rotation"}, {"Activ"=FALSE, "X"=90.0, "Y"=0.0, "Z"=0.0, "Div"=0, "Set 1"=FALSE, "Set 2"=FALSE, "Set 3"=FALSE, "Skip"=FALSE, "action"=enum."Rotation"}, {"Activ"=FALSE, "X"=90.0, "Y"=0.0, "Z"=0.0, "Div"=0, "Set 1"=FALSE, "Set 2"=FALSE, "Set 3"=FALSE, "Skip"=FALSE, "action"=enum."Rotation"}, {"Activ"=FALSE, "X"=1.0, "Y"=0.0, "Z"=0.0, "Div"=0, "Set 1"=FALSE, "Set 2"=FALSE, "Set 3"=FALSE, "Skip"=FALSE, "action"=enum."Smooth pause"}, {"Activ"=FALSE, "X"=90.0, "Y"=0.0, "Z"=0.0, "Div"=0, "Set 1"=FALSE, "Set 2"=FALSE, "Set 3"=FALSE, "Skip"=FALSE, "action"=enum."Rotation Correct"}]
  in  "Array 27":T3(array[cluster])
  in  "LED Green":bool
  in  "LED Red":bool
  in  "Blink Green":bool
  in  "Blink Red":bool
  in  "Tab Plate":enum32{"Movement&OMS", "Camera", "Joystick"}(tab)
  out "wall stop":bool
  in  "ServoA":dbl[](array[numeric])=[32.0, 25.0]
  in  "Speed":dbl=95.0
  in  "upper limit":cluster{"X":dbl, "Y":dbl, "Z":dbl}={"X"=0.8, "Y"=0.8, "Z"=0.5}
  out "Tab True":T4 items=["Script 0", "Script 1", "Script 2", "Script 3", "Script 4", "Script 5", "Script 6", "Script 7", "Script 8", "Script 9", "Script 10", "Script 11", "Script 12", "Script 13", "Script 14", "Script 15", "Script 16", "Script 17", "Script 18", "Script 19", "Script 20", "Script 21", "Script 22", "Script 23", "Script 24", "Script 25", "Script 26", "Script 27"]
  in  "Lift Level":dbl=5.0
  in  "Lift parameters":T5={"Limit L"=0.0, "Limit H"=34.0, "Ratio"=0.00344}
  out "ENC":T6
  out "M Lift":dbl
  out "Lift":dbl(slide) scale=0.0..35.0
  out "Lift in  Range":bool
  in  "Lift Reset":bool
  in  "Motors Renum":cluster{"Num":i32, "Directly":bool, "KM":dbl}[](array[cluster])=[{"Num"=0, "Directly"=TRUE, "KM"=1.05}, {"Num"=1, "Directly"=FALSE, "KM"=1.0}, {"Num"=2, "Directly"=FALSE, "KM"=0.95}, {"Num"=3, "Directly"=TRUE, "KM"=1.0}]
  out "Motors":T7 {"M Back" format="%#_4g"; "M Right" format="%#_4g"; "M Left" format="%#_4g"}
  in  "PID gains":T8={"proportional gain (Kc)"=0.95, "integral time (Ti, min)"=0.01, "derivative time (Td, min)"=0.0} {"derivative time (Td, min)" format="%.3f"; "integral time (Ti, min)" format="%.3f"; "proportional gain (Kc)" format="%.3f"}
  in  "Break":bool
  in  "Reset Enc":bool
  out "ENC True":T6
  out "RPM":T9
  in  "Factor":cluster{"Kx":dbl, "Kz":dbl, "Ky":dbl}={"Kx"=0.02114, "Kz"=0.0705, "Ky"=0.0245} {"Ky" format="%#_13g"; "Kz" format="%#_13g"; "Kx" format="%#_13g"}
  in  "Servo":dbl=26.0 min=0.0 max=255.0 step=1.0
  out "IR":cluster{"IR Left":dbl, "IR Right":dbl}
  out "PING":cluster{"PING left":dbl, "PING right":dbl}
  out "move ind":dbl
  out "X":dbl
  out "Y":dbl
  out "IR median":dbl
  out "YAW (degree)":dbl
  in  "Array Null":T3(array[cluster])
  out "QTI Binary Custom":bool[](array[boolean])
  out "YAW (degree) 2":dbl
  in  "Array":enum8{"R1", "R2", "R3", "R4", "R5", "NS"}[](array[ring])=[enum."R1", enum."R2", enum."R3", enum."R4", enum."R5", enum."NS"]
  in  "Order Board":dbl[][](array[ring])=[[0.0, 0.0, 0.0, 0.0, 0.0, 0.0], [0.0, 0.0, 0.0, 0.0, 0.0, 0.0], [1.0, 2.0, 0.0, 0.0, 0.0, 0.0], [0.0, 4.0, 0.0, 0.0, 0.0, 0.0], [0.0, 0.0, 0.0, 0.0, 0.0, 0.0], [0.0, 0.0, 0.0, 0.0, 0.0, 0.0]]
  in  "Camera result":string
  out "String to array":dbl[](array[numeric])
  out "Action":dbl
  out "Div":i8
  out "x-y":dbl
  out "s? t:f":dbl
  out "element":dbl
  in  "index":i32
  out "size(s)":i32
  out "Joystick":T10={"L Stick"=FALSE, "R Stick"=FALSE, "X"=FALSE, "A"=FALSE, "Y"=FALSE, "B"=FALSE, "45"=FALSE, "90"=FALSE, "135"=FALSE, "180"=FALSE, "225"=FALSE, "270"=FALSE, "315"=FALSE, "0"=FALSE, "Start"=FALSE, "Back"=FALSE, "RB"=FALSE, "LB"=FALSE, "X Right"=0, "Y Right"=0, "X Left"=0, "Y Left"=0, "Z Right"=0, "Pov"=-1, "Z Left"=0, "Num"=0} {"Z Right" scale=0.0..100.0; "Y Left" scale=-100.0..100.0; "X Left" scale=-100.0..100.0; "Y Right" scale=-100.0..100.0; "X Right" scale=-100.0..100.0}
  out "coerced(x)":dbl
  out "X Right":i8
  out "Y Right":i8
  in  "Start Button":bool
  in  "Stop Button":bool
  # "1 = 0.36 мм    83 = ~90*"
  # "Скрипт 20 - старт, фото, скан доски."
  # "Скрипт 21 - ехать в комнату 1"
  # "Скрипт 2- №1 ОСТАНОВКА ПО ДАТЧИКУ"
  # "Скрипт 22 - ехать в комнату 2"
  # "Скрипт 3- №2 ДЕЗИНФЕКЦИЯ"
  # "Скрипт 23 - ехать в комнату 3"
  # "Скрипт 20- №8 КАМЕРА"
  # "Скрипт 24 - ехать в комнату 4"
  # "Скрипт 25 - ехать в комнату 5"
  # "Скрипт 26 - ехать в комнату NS"
  # "При вращении надо ставить угол на 7 градусов меньше!!!"
  # "Control"
  # "GPS"
  # "X\n\nY\n\nZ"
  # "ТОЛЬКО для отображения выполнения программы!"
  # "Место для коментария скрипта.\n                Команда         X      Y     Z   Div 1  2  3  Off"
  # "Место для коментария скрипта.\n                Команда         X      Y     Z   Div 1  2  3  Off"
  # "Место для коментария скрипта.\n                Команда         X      Y     Z   Div 1  2  3  Off"
  # "Место для коментария скрипта.\n                Команда         X      Y     Z   Div 1  2  3  Off"
  # "Место для коментария скрипта.\n                Команда         X      Y     Z   Div 1  2  3  Off"
  # "Место для коментария скрипта.\n                Команда         X      Y     Z   Div 1  2  3  Off"
  # "Место для коментария скрипта.\n                Команда         X      Y     Z   Div 1  2  3  Off"
  # "Место для коментария скрипта.\n                Команда         X      Y     Z   Div 1  2  3  Off"
  # "Место для коментария скрипта.\n                Команда         X      Y     Z   Div 1  2  3  Off"
  # "Место для коментария скрипта.\n                Команда         X      Y     Z   Div 1  2  3  Off"
  # "Место для коментария скрипта.\n                Команда         X      Y     Z   Div 1  2  3  Off"
  # "Место для коментария скрипта.\n                Команда         X      Y     Z   Div 1  2  3  Off"
  # "Место для коментария скрипта.\n                Команда         X      Y     Z   Div 1  2  3  Off"
  # "Место для коментария скрипта.\n                Команда         X      Y     Z   Div 1  2  3  Off"
  # "Место для коментария скрипта.\n                Команда         X      Y     Z   Div 1  2  3  Off"
  # "Место для коментария скрипта.\n                Команда         X      Y     Z   Div 1  2  3  Off"
  # "Место для коментария скрипта.\n                Команда         X      Y     Z   Div 1  2  3  Off"
  # "Место для коментария скрипта.\n                Команда         X      Y     Z   Div 1  2  3  Off"
  # "Место для коментария скрипта.\n                Команда         X      Y     Z   Div 1  2  3  Off"
  # "Место для коментария скрипта.\n                Команда         X      Y     Z   Div 1  2  3  Off"
  # "Место для коментария скрипта.\n                Команда         X      Y     Z   Div 1  2  3  Off"
  # "Место для коментария скрипта.\n                Команда         X      Y     Z   Div 1  2  3  Off"
  # "Место для коментария скрипта.\n                Команда         X      Y     Z   Div 1  2  3  Off"
  # "Место для коментария скрипта.\n                Команда         X      Y     Z   Div 1  2  3  Off"
  # "Место для коментария скрипта.\n                Команда         X      Y     Z   Div 1  2  3  Off"
  # "Место для коментария скрипта.\n                Команда         X      Y     Z   Div 1  2  3  Off"
  # "Место для коментария скрипта.\n                Команда         X      Y     Z   Div 1  2  3  Off"
  # "PID"
  # "Movement"
  # "Геймпад во 2 скрипте"
  # "Левый"
  # "X\n\nY\n\nZ"
  # "Правый"
  # "Задний"
  # "Лифт"
  # "OMS"
  # "D\nE\nL\nI\nV\nE\nR"
  # "R\nE\nT"
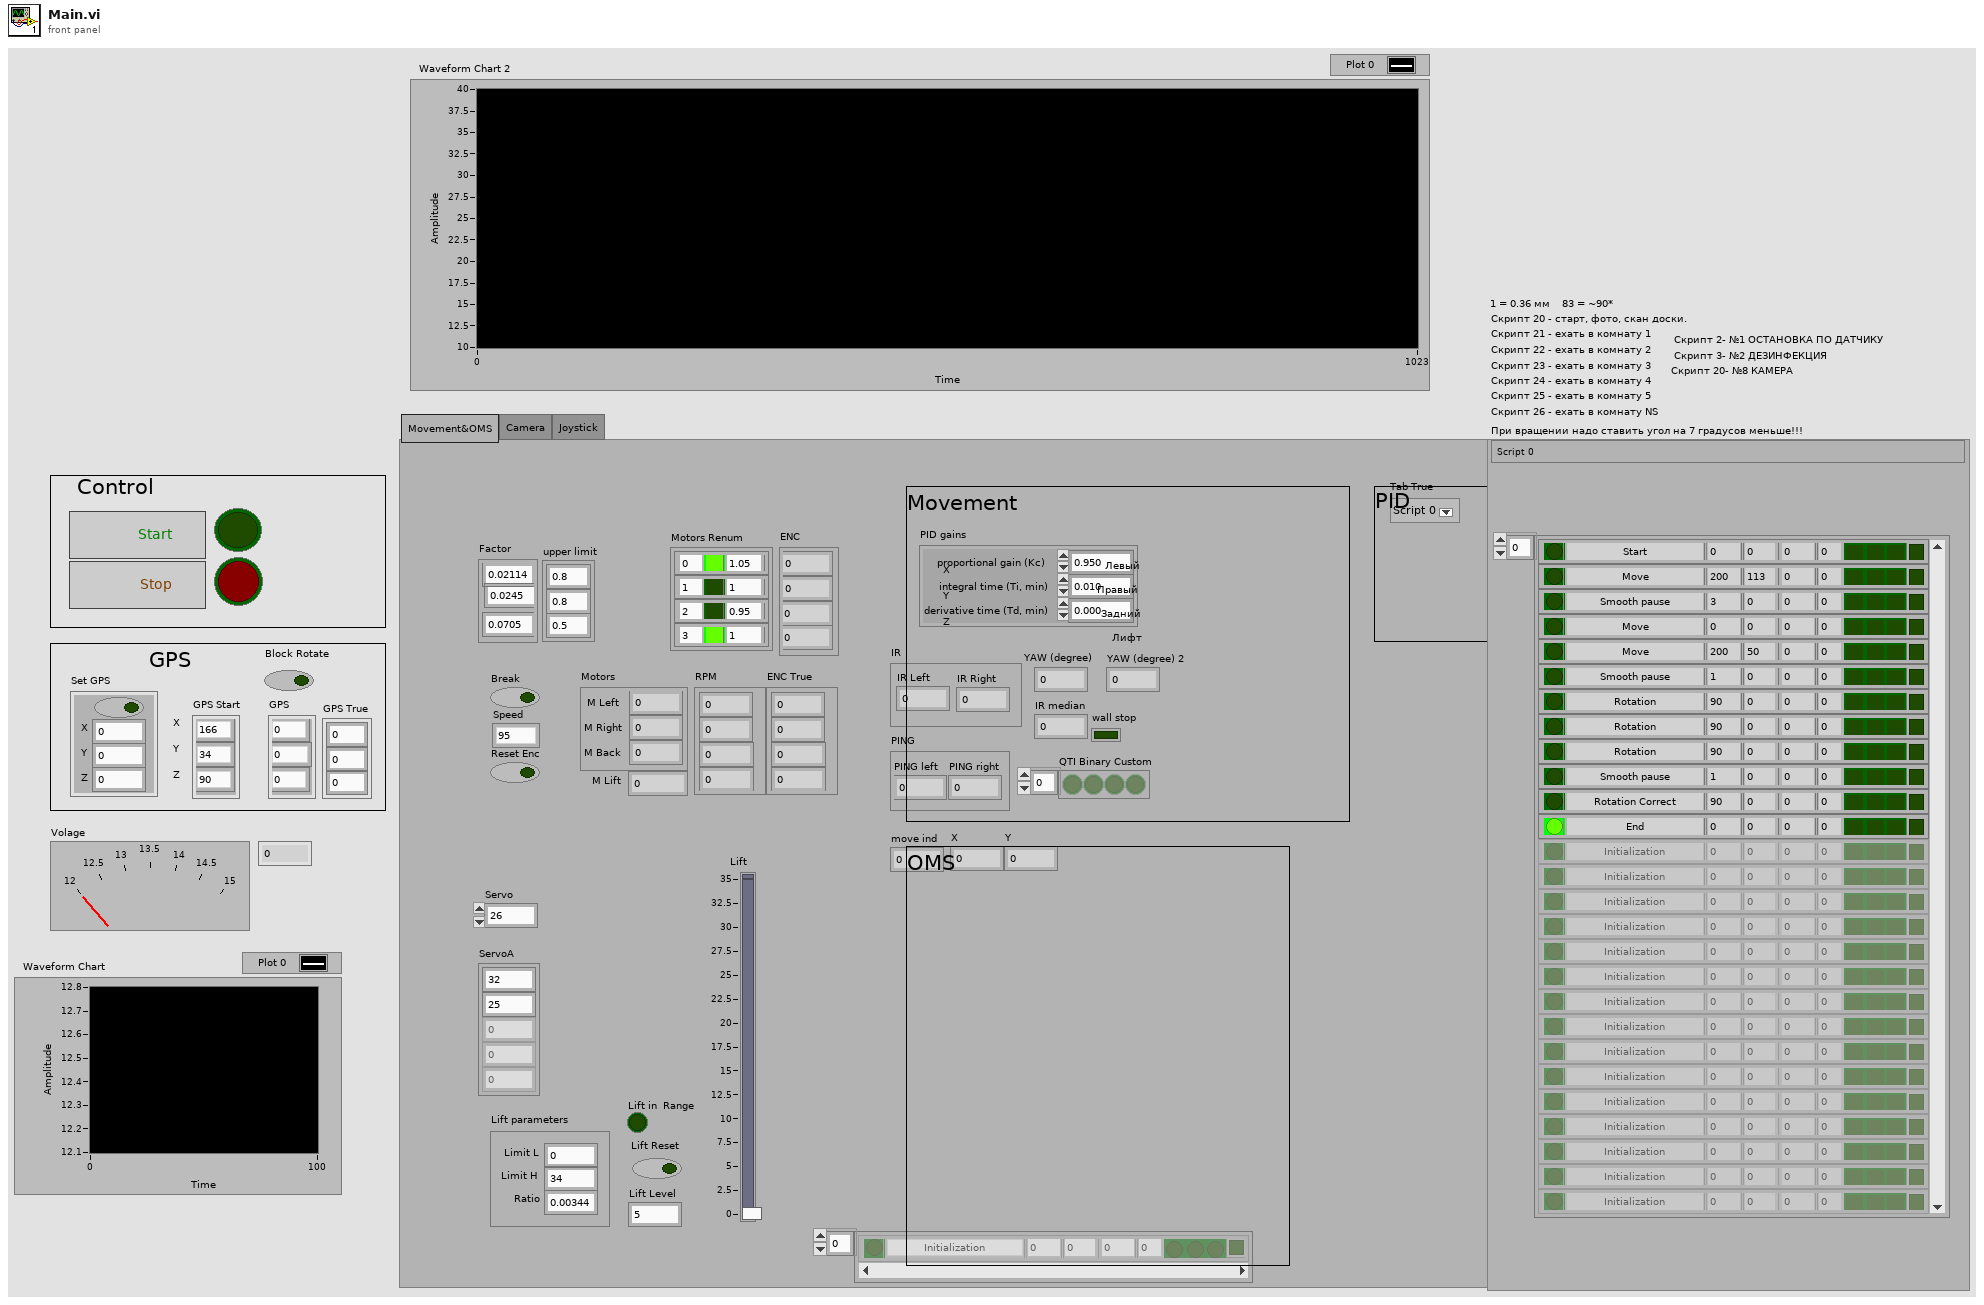
[diagram p1: front panel]
types:
  T1 = enum32{"Script 0", "Script 1", "Script 2", "Script 3", "Script 4", "Script 5", "Script 6", "Script 7", "Script 8", "Script 9", "Script 10", "Script 11", "Script 12", "Script 13", "Script 14", "Script 15", "Script 16", "Script 17", "Script 18", "Script 19", "Script 20", "Script 21", "Script 22", "Script 23", "Script 24", "Script 25", "Script 26", "Script 27"}
  T2 = typedef "Action control.ctl" = enum16{"Initialization", "Start", "Smooth pause", "autonomus", "Pause", "Camera", "Rotation", "Rotation Correct", "Move", "Move GPS", "Lift", "OMS", "Gamepad", "Go to", "Empty script", "Run scripts", "End"}
  T3 = cluster{"Activ":bool, "X":dbl, "Y":dbl, "Z":dbl, "Div":i8, "Set 1":bool, "Set 2":bool, "Set 3":bool, "Skip":bool, "action":T2}[]
  T4 = typedef "Script control.ctl" = u32
  T5 = cluster{"Limit L":dbl, "Limit H":dbl, "Ratio":dbl}
  T6 = cluster{"ENC Left":i32, "ENC Right":i32, "ENC Back":i32, "ENC Lift":i32}
  T7 = cluster{"M Left":dbl, "M Right":dbl, "M Back":dbl}
  T8 = cluster{"proportional gain (Kc)":dbl, "integral time (Ti, min)":dbl, "derivative time (Td, min)":dbl}
  T9 = cluster{"RPM Left":i32, "RPM Right":i32, "RPM Back":i32, "RPM Lift":i32}
  T10 = typedef "Joystick controls.ctl" = cluster{"L Stick":bool, "R Stick":bool, "X":bool, "A":bool, "Y":bool, "B":bool, "45":bool, "90":bool, "135":bool, "180":bool, "225":bool, "270":bool, "315":bool, "0":bool, "Start":bool, "Back":bool, "RB":bool, "LB":bool, "X Right":i8, "Y Right":i8, "X Left":i8, "Y Left":i8, "Z Right":i8, "Pov":i16, "Z Left":i8, "Num":i16}
  T11 = typedef "XDNodeRunTimeDep.lvlib/timing_clust.ctl" = cluster{"Expected End [f-1]":u64, "Actual End [f-1]":u64, "Finished Late? [f-1]":bool, "Expected End [i-1]":u64, "Actual End [i-1]":u64, "Finished Late? [i-1]":bool, "Expected Start [i]":u64, "Actual Start [i]":u64, "Expected Start [f]":u64, "Actual Start [f]":u64, "Source Name":string, "Structure Name":string, "Period":i64, "Deadline":i64, "Offset":i64, "Start":i64, "Priority":i32, "Timeout":i32, "Mode":T12, "Wakeup Reason":T13, "Error":errorcluster, "Source Type":string, "Secondary Source Type":string, "Global End Time":u64, "Global Start Time":u64, "Frame Duration":u64, "Iteration Duration":u64, "Assigned CPU":i32, "I/O Scan Engine Mode":u32}
  T12 = typedef "XDNodeRunTimeDep.lvlib/nitl_modes.ctl" = enum32{"No Change", "Process missed periods, maintain original phase", "Discard missed periods, maintain original phase", "Process missed periods, ignore original phase", "Discard missed periods, ignore original phase"}
  T13 = typedef "XDNodeRunTimeDep.lvlib/wakeup.ctl" = enum32{"Normal", "Aborted", "Asynchronous wakeup", "Timing source error", "Timed loop error", "Timeout"}
  T14 = cluster{"Enc Left":i32, "Enc Right":i32, "Enc Back":i32}
  T15 = cluster{"Limit H":refnum<class "Digital Input and Output.lvclass">, "Limit L":refnum<class "Digital Input and Output.lvclass">}
  T16 = cluster{"Button Start":refnum<class "Digital Input and Output.lvclass">, "Button Stop":refnum<class "Digital Input and Output.lvclass">}
  T17 = cluster{"LED Red":refnum<class "Digital Input and Output.lvclass">, "LED Green":refnum<class "Digital Input and Output.lvclass">}
  T18 = cluster{"Analog":refnum<class "Analog In.lvclass">, "Voltage":refnum<class "Analog In.lvclass">}
  T19 = cluster{"Ir Sensor L":refnum<class "Analog In.lvclass">, "Ir Sensor R":refnum<class "Analog In.lvclass">}
  T20 = cluster{"Puls L":refnum<class "Pulse.lvclass">, "Eсho L":refnum<class "ISQ.lvclass">, "Puls R":refnum<class "Pulse.lvclass">, "Eсho R":refnum<class "ISQ.lvclass">}
  T21 = cluster{"TitanENC 0":refnum<class "TitanENC.lvclass">, "TitanENC 1":refnum<class "TitanENC.lvclass">, "TitanENC 2":refnum<class "TitanENC.lvclass">, "TitanENC 3":refnum<class "TitanENC.lvclass">}
  T22 = cluster{"Ir Sensor":cluster{"Ir Sensor L":refnum<class "Analog In.lvclass">, "Ir Sensor R":refnum<class "Analog In.lvclass">}, "Ultrasonic":cluster{"Puls L":refnum<class "Pulse.lvclass">, "Eсho L":refnum<class "ISQ.lvclass">, "Puls R":refnum<class "Pulse.lvclass">, "Eсho R":refnum<class "ISQ.lvclass">}, "Line Sensor":refnum<class "IIC.lvclass">, "DC Motors":refnum<class "CAN.lvclass">, "TitanENC":cluster{"TitanENC 0":refnum<class "TitanENC.lvclass">, "TitanENC 1":refnum<class "TitanENC.lvclass">, "TitanENC 2":refnum<class "TitanENC.lvclass">, "TitanENC 3":refnum<class "TitanENC.lvclass">}, "Switch":cluster{"Limit H":refnum<class "Digital Input and Output.lvclass">, "Limit L":refnum<class "Digital Input and Output.lvclass">}, "Buttons":cluster{"Button Start":refnum<class "Digital Input and Output.lvclass">, "Button Stop":refnum<class "Digital Input and Output.lvclass">}, "LEDs":cluster{"LED Red":refnum<class "Digital Input and Output.lvclass">, "LED Green":refnum<class "Digital Input and Output.lvclass">}, "Servo":refnum<class "PWM.lvclass">, "Analog":cluster{"Analog":refnum<class "Analog In.lvclass">, "Voltage":refnum<class "Analog In.lvclass">}, "Gyroscope":refnum<class "IMU.lvclass">}
  T23 = cluster{"Activ":bool, "X":dbl, "Y":dbl, "Z":dbl, "Div":i8, "Set 1":bool, "Set 2":bool, "Set 3":bool, "Skip":bool, "action":T2}
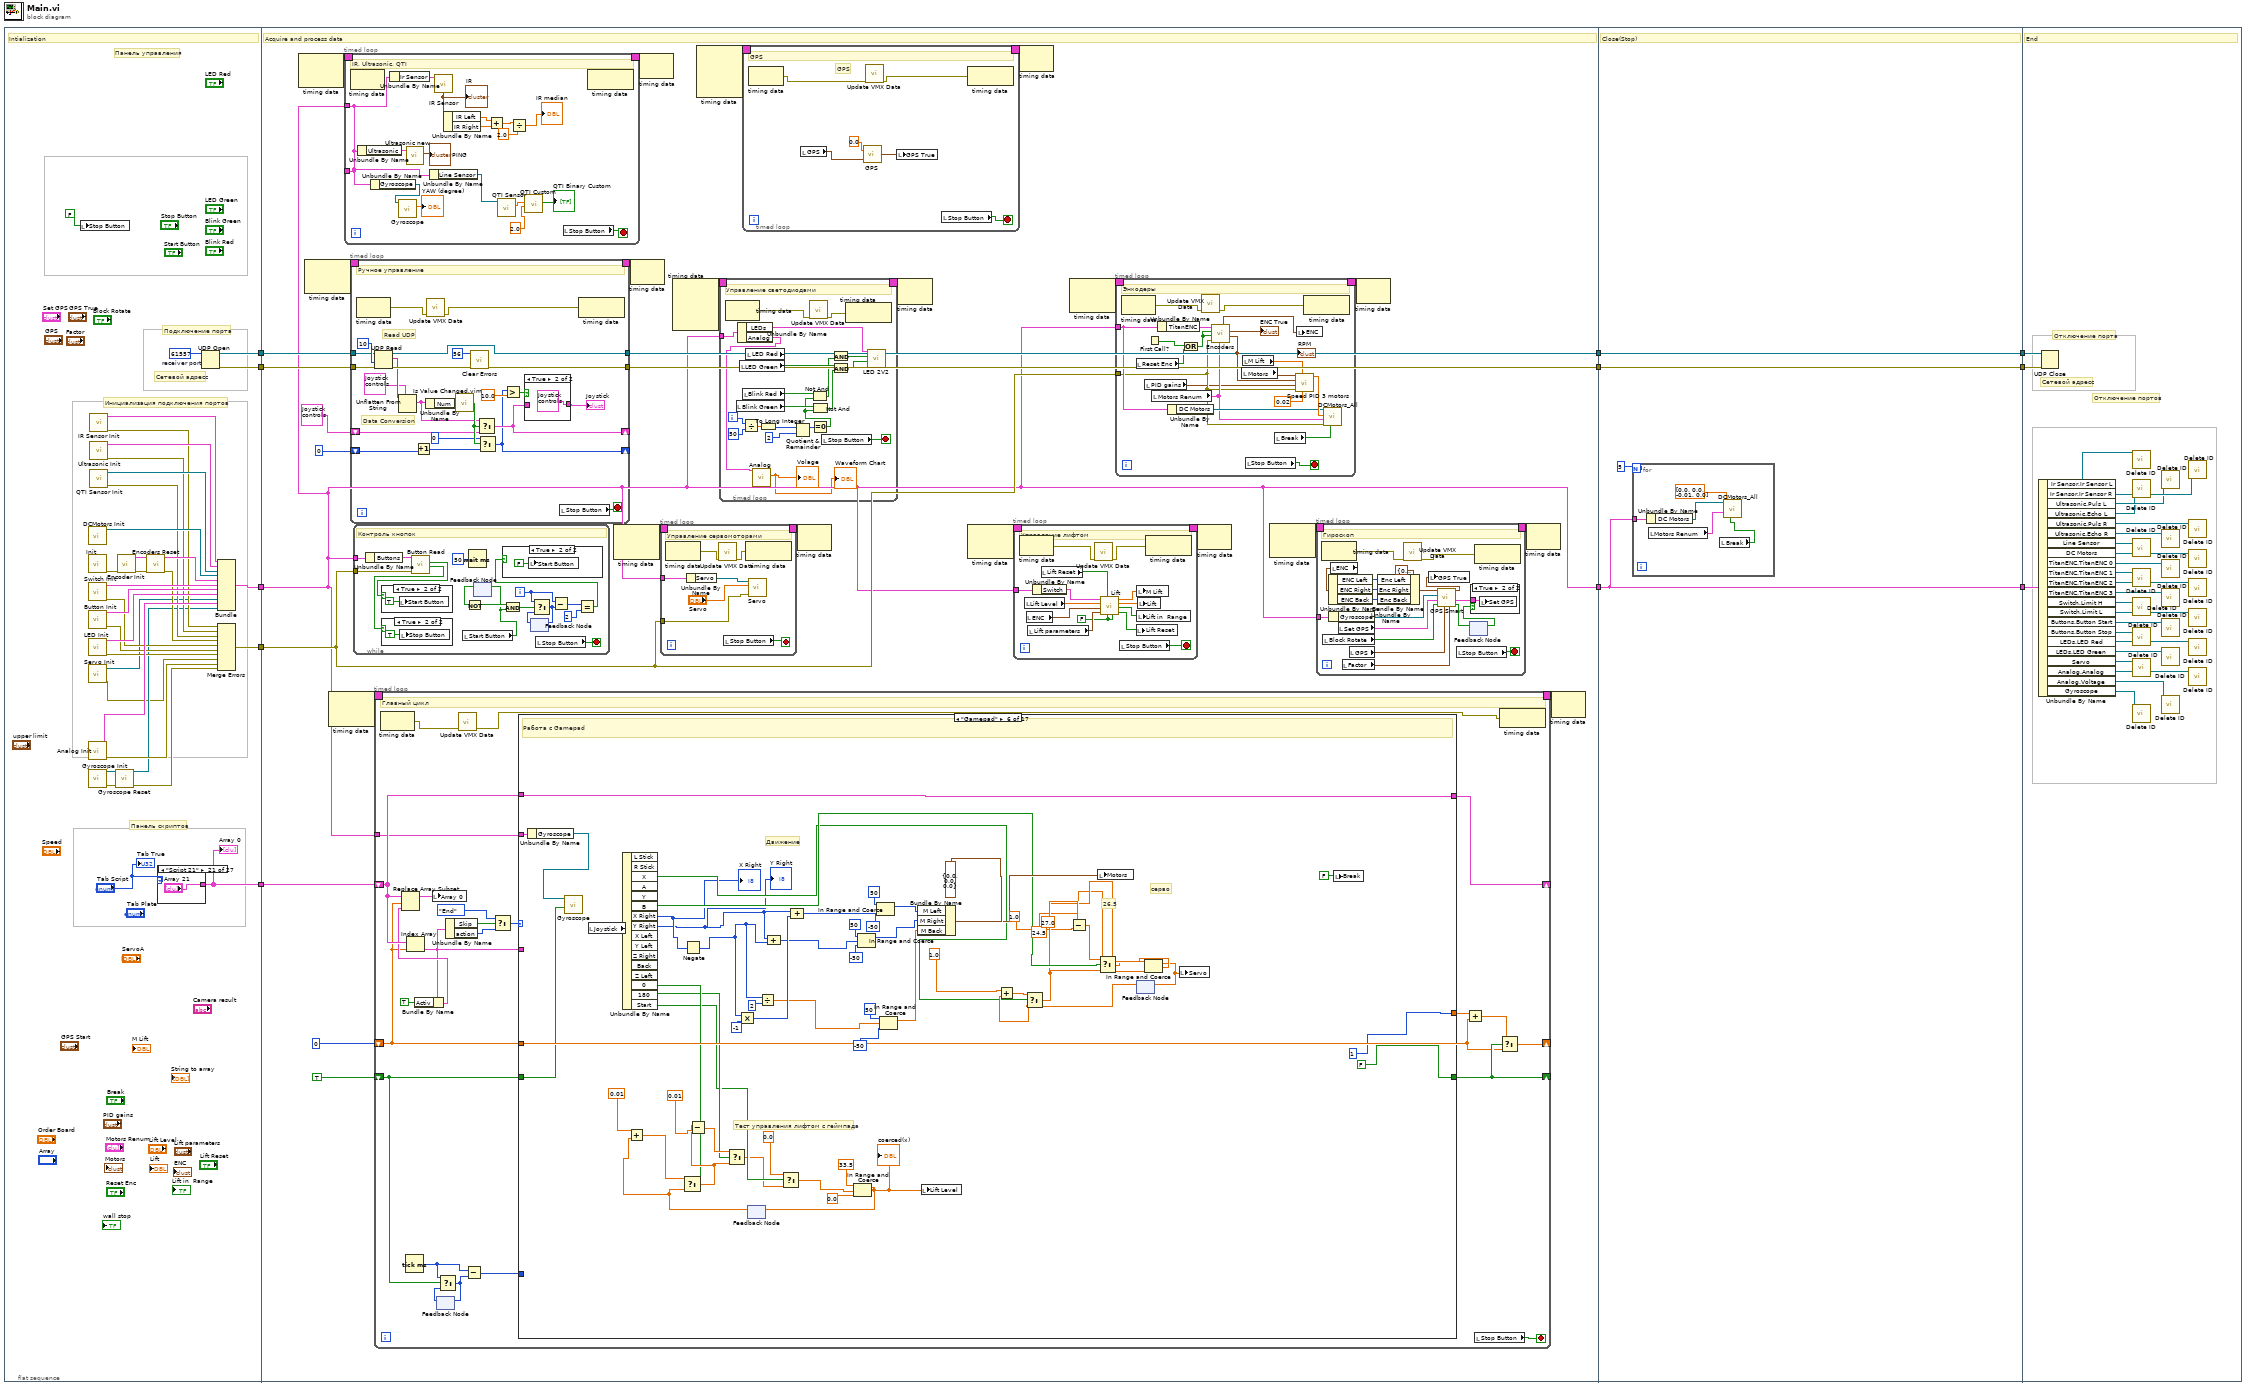
[diagram p0: block diagram]
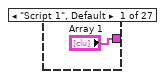
[diagram p2: hidden frame]
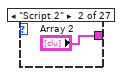
[diagram p3: hidden frame]
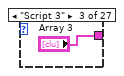
[diagram p4: hidden frame]
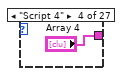
[diagram p5: hidden frame]
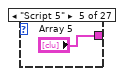
[diagram p6: hidden frame]
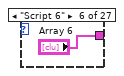
[diagram p7: hidden frame]
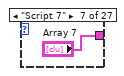
[diagram p8: hidden frame]
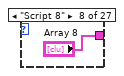
[diagram p9: hidden frame]
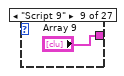
[diagram p10: hidden frame]
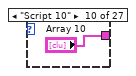
[diagram p11: hidden frame]
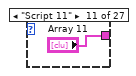
[diagram p12: hidden frame]
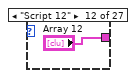
[diagram p13: hidden frame]
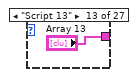
[diagram p14: hidden frame]
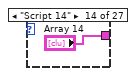
[diagram p15: hidden frame]
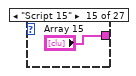
[diagram p16: hidden frame]
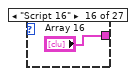
[diagram p17: hidden frame]
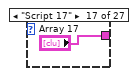
[diagram p18: hidden frame]
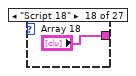
[diagram p19: hidden frame]
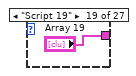
[diagram p20: hidden frame]
diagram:
  n1 = flat-sequence {
    tunnel: [w24] -> w9
    tunnel: [w23] -> w6
    tunnel: [w22] -> w3
    tunnel: [w20] -> w2
    tunnel: [w14] -> w1
    tunnel: [w73] -> w10
    tunnel: w9 -> [w73]
    tunnel: [w97] -> w7
    tunnel: w6 -> [w99]
    tunnel: [w96] -> w4
    tunnel: w3 -> [w98]
    tunnel: w2 -> [w81]
    tunnel: w1 -> [w88]
    tunnel: [w770] -> w11
    tunnel: w10 -> [w770]
    tunnel: [w773] -> w8
    tunnel: w7 -> [w773]
    tunnel: [w772] -> w5
    tunnel: w4 -> [w772]
    tunnel: w11 -> [w803]
    tunnel: w8 -> [w781]
    tunnel: w5 -> [w780]
    frame #0 {
      w45 = u16 61557  # receiver port
      # "Панель скриптов"
      # "Панель управления"
      # "Инициализация подключения портов"
      # "Подключение порта"
      # "Сетевой адресс"
      # "Intialization"
      n2 = local write "Stop Button"(FALSE ("Stop Button")) -> ()
      n3 = call "DCMotors Init.vi"() -> ("DC Motors"=w41:refnum<class "CAN.lvclass">)  [unwired: 10 in, 1 out]
      n4 = call <vilib>:"Init.vi"() -> ("error out"=w40:errorcluster)  [unwired: 11 in]
      n5 = call "Switch Init.vi"() -> ("error out"=w28:errorcluster, "Switch"=w36:T15)  [unwired: 10 in]
      n6 = call "Button Init.vi"() -> ("error out"=w27:errorcluster, "Buttons"=w35:T16)  [unwired: 10 in]
      n7 = call "LED Init.vi"() -> ("error out"=w26:errorcluster, "LEDs"=w34:T17)  [unwired: 10 in]
      n8 = call "Servo Init.vi"() -> ("error out"=w12:errorcluster, "Servo"=w13:refnum<class "PWM.lvclass">)  [unwired: 10 in]
      n9 = call "Analog Init.vi"() -> ("error out"=w25:errorcluster, "Analog"=w33:T18)  [unwired: 10 in]
      n10 = call "Gyroscope Init.vi"() -> ("error out"=w18:errorcluster, "Gyroscope"=w19:refnum<class "IMU.lvclass">)  [unwired: 10 in]
      n11 = call "IR Sensor Init.vi"() -> ("error out"=w32:errorcluster, "Ir Sensor"=w44:T19)  [unwired: 10 in]
      n12 = call "Ultrasonic Init.vi"() -> ("error out"=w31:errorcluster, "Ultrasonic"=w43:T20)  [unwired: 10 in]
      n13 = call "QTI Sensor Init.vi"() -> ("error out"=w30:errorcluster, "Line Sensor"=w42:refnum<class "IIC.lvclass">)  [unwired: 10 in]
      n14 = call "Gyroscope Reset.vi"("error in (no error)"=w18, "Gyroscope in"=w19) -> ("error out"=w16:errorcluster, "Gyroscope"=w17:refnum<class "IMU.lvclass">)  [unwired: 8 in]
      n15 = call "Encoder Init.vi"("error in (no error)"=w40) -> ("error out"=w39:errorcluster, "TitanENC out"=w38:T21)  [unwired: 9 in]
      n16 = call "Encoders Reset.vi"("error in (no error)"=w39, "TitanENC in"=w38) -> ("error out"=w29:errorcluster, "TitanENC"=w37:T21)  [unwired: 8 in]
      n17 = case shown="\"Script 21\"" "Tab Script" {
        tunnel: ["Array 1" "Array 2" "Array 3" "Array 4" "Array 5" "Array 6" "Array 7" "Array 8" "Array 9" "Array 10" "Array 11" "Array 12" "Array 13" "Array 14" "Array 15" "Array 16" "Array 17" "Array 18" "Array 19" "Array 20" "Array 21" "Array 22" "Array 23" "Array 24" "Array 25" "Array 26" "Array 27"] -> w14
        frame "Script 1", Default {
        }
        frame "Script 2" {
        }
        frame "Script 3" {
        }
        frame "Script 4" {
        }
        frame "Script 5" {
        }
        frame "Script 6" {
        }
        frame "Script 7" {
        }
        frame "Script 8" {
        }
        frame "Script 9" {
        }
        frame "Script 10" {
        }
        frame "Script 11" {
        }
        frame "Script 12" {
        }
        frame "Script 13" {
        }
        frame "Script 14" {
        }
        frame "Script 15" {
        }
        frame "Script 16" {
        }
        frame "Script 17" {
        }
        frame "Script 18" {
        }
        frame "Script 19" {
        }
        frame "Script 20" {
        }
        frame "Script 21" {
        }
        frame "Script 22" {
        }
        frame "Script 23" {
        }
        frame "Script 24" {
        }
        frame "Script 25" {
        }
        frame "Script 26" {
        }
        frame "Script 27" {
        }
      }
      "Array 0" <- w14
      n18 = UDP Open(11:w45) -> (port=w23:refnum<k16>, 0:w22:errorcluster)  [unwired: 4 in, 1 out]
      n19 = Bundle("Ir Sensor"=w44, "Ultrasonic"=w43, "Line Sensor"=w42, "DC Motors"=w41, "TitanENC"=w37, "Switch"=w36, "Buttons"=w35, "LEDs"=w34, "Servo"=w13, "Analog"=w33, "Gyroscope"=w17) -> (w24:T22)  [unwired: 1 in]
      n20 = Merge Errors(w32, w31, w30, w29, w28, w27, w26, w12, w25, w16) -> (w20:errorcluster)
      "Tab True" <- "Tab Script"
    }
    frame #1 {
      # "Acquire and process data"
      n21 = node-c288() -> (w79:T11)  [unwired: 2 in]
      n22 = node-c288() -> (w101:T11)  [unwired: 2 in]
      n23 = node-c288() -> (w77:T11)  [unwired: 2 in]
      n24 = timed-loop {
        timing: w79 -> [_]
        timing-out: [_] -> w78
        tunnel: w73 -> [w579]
        tunnel: [w579] -> _
        stop <- w594 stop-if-true
        # "IR, Ultrasonic, QTI"
        n25 = node-c288() -> ()  [unwired: 1 in, 1 out]
        n26 = Unbundle By Name(w579) -> ("Ultrasonic"=w592:T20)
        n27 = Unbundle By Name(w579) -> ("Gyroscope"=w584:refnum<class "IMU.lvclass">)
        n28 = Unbundle By Name(w579) -> ("Ir Sensor"=w593:T19)
        n29 = call "Gyroscope.vi"("IMU in"=w584) -> ("YAW (degree)"=→"YAW (degree)":dbl)  [unwired: 6 in, 4 out]
        n30 = call "Ultrasonic new.vi"("Pulse in"=w592) -> ("PING"=→"PING":cluster{"PING left":dbl, "PING right":dbl})  [unwired: 8 in, 2 out]
        n31 = Unbundle By Name(w579) -> ("Line Sensor"=w580:refnum<class "IIC.lvclass">)
        n32 = call "IR Sensor.vi"("Analog In in"=w593) -> ("IR"=w590:cluster{"IR Left":dbl, "IR Right":dbl})  [unwired: 8 in, 2 out]
        "IR" <- w590
        n33 = Unbundle By Name(w590) -> ("IR Left"=w588:dbl, "IR Right"=w589:dbl)
        n34 = Add(x=w588, y=w589) -> (x+y=w587:dbl)
        n35 = call "QTI Sensor.vi"("IIC in"=w580) -> ("QTI"=w581:dbl[])  [unwired: 7 in, 3 out]
        n36 = Divide(x=w587, y=2.0) -> (x/y=→"IR median":dbl)
        n37 = call "QTI Custom.vi"("num"=2.0, "QTI Raw"=w581) -> ("QTI Binary Custom"=→"QTI Binary Custom":bool[])  [unwired: 8 in, 1 out]
        n38 = local read "Stop Button"() -> (w594:bool)
        n39 = node-c288() -> ()  [unwired: 1 in, 1 out]
      }
      n40 = timed-loop {
        timing: w101 -> [_]
        timing-out: [_] -> w100
        tunnel: w99 -> [w756]
        tunnel: w98 -> [w755]
        tunnel: [w753] -> w97
        tunnel: [w752] -> w96
        shift-right: [w740] -> _
        shift-left: 0 ("specific error code to clear (0: all)") -> [w747]
        shift-right: [w742] -> _
        shift-left: T10 {"L Stick"=FALSE, "R Stick"=FALSE, "X"=FALSE, "A"=FALSE, "Y"=FALSE, "B"=FALSE, "45"=FALSE, "90"=FALSE, "135"=FALSE, "180"=FALSE, "225"=FALSE, "270"=FALSE, "315"=FALSE, "0"=FALSE, "Start"=FALSE, "Back"=FALSE, "RB"=FALSE, "LB"=FALSE, "X Right"=0, "Y Right"=0, "X Left"=0, "Y Left"=0, "Z Right"=0, "Pov"=-1, "Z Left"=0, "Num"=0} ("Joystick") -> [w743]
        stop <- w739 stop-if-true
        # "Data Conversion"
        # "Read UDP"
        # "Ручное управление"
        n41 = node-c288() -> (w760:errorcluster)  [unwired: 1 in]
        n42 = UDP Read(connection ID=w756, timeout ms (25000)=10, 8:w755) -> (data out=w745:string, error out=w754:errorcluster, 3:w753:refnum<k16>)  [unwired: 1 in, 2 out]
        n43 = Unflatten From String(type=T10 {"L Stick"=FALSE, "R Stick"=FALSE, "X"=FALSE, "A"=FALSE, "Y"=FALSE, "B"=FALSE, "45"=FALSE, "90"=FALSE, "135"=FALSE, "180"=FALSE, "225"=FALSE, "270"=FALSE, "315"=FALSE, "0"=FALSE, "Start"=FALSE, "Back"=FALSE, "RB"=FALSE, "LB"=FALSE, "X Right"=0, "Y Right"=0, "X Left"=0, "Y Left"=0, "Z Right"=0, "Pov"=-1, "Z Left"=0, "Num"=0} ("Joystick"), binary string=w745) -> (value=w744:T10)  [unwired: 3 in, 2 out]
        n44 = Increment(x=w747) -> (x+1=w750:i32)
        n45 = Unbundle By Name(w744) -> ("Num"=w746:i16)
        n46 = call <vilib>:"Update VMX Data.vi"("error in (no error)"=w760) -> ("error out"=w759:errorcluster)  [unwired: 10 in]
        n47 = call "Is Value Changed.vim"("value"=w746) -> ("changed or first call?"=w749:bool)
        n48 = call <vilib>:"Clear Errors.vi"("error in (no error)"=w754, "specific error code to clear (0: all)"=56) -> ("error out"=w752:errorcluster)  [unwired: 4 in, 1 out]
        n49 = Select(t=w744, s=w749, f=w743) -> (s? t:f=w742:T10)
        n50 = Select(t=0 ("specific error code to clear (0: all)"), s=w749, f=w750) -> (s? t:f=w740:i32)
        n51 = Greater?(x=w740, y=10.0) -> (0:w741:bool)
        n52 = case shown="True" w741 {
          tunnel: [w761 T10 {"L Stick"=FALSE, "R Stick"=FALSE, "X"=FALSE, "A"=FALSE, "Y"=FALSE, "B"=FALSE, "45"=FALSE, "90"=FALSE, "135"=FALSE, "180"=FALSE, "225"=FALSE, "270"=FALSE, "315"=FALSE, "0"=FALSE, "Start"=FALSE, "Back"=FALSE, "RB"=FALSE, "LB"=FALSE, "X Right"=0, "Y Right"=0, "X Left"=0, "Y Left"=0, "Z Right"=0, "Pov"=-1, "Z Left"=0, "Num"=0} ("Joystick")] -> w738
          tunnel: w742 -> [w761 _]
          frame False {
          }
          frame True {
          }
        }
        "Joystick" <- w738
        n53 = local read "Stop Button"() -> (w739:bool)
        n54 = node-c288(w759) -> ()  [unwired: 1 out]
      }
      n55 = while {
        tunnel: w73 -> [w732]
        tunnel: w81 -> [w717]
        i -> [w722]
        stop <- w733 stop-if-true
        # "Контроль кнопок"
        n56 = Unbundle By Name(w732) -> ("Buttons"=w731:T16)
        n57 = call "Button Read.vi"("error in (no error)"=w717, "HG_LIB in"=w731) -> ("Stop"=w729:bool, "Start"=w730:bool)  [unwired: 6 in, 2 out]
        n58 = case shown="True" w730 {
          frame False {
          }
          frame True {
            n59 = local write "Start Button"(TRUE ("Start Button")) -> ()
          }
        }
        n60 = case shown="True" w729 {
          frame False {
          }
          frame True {
            n61 = local write "Stop Button"(TRUE ("Start Button")) -> ()
          }
        }
        n62 = local read "Start Button"() -> (w721:bool)
        n63 = Wait (ms)(milliseconds to wait=u32 50) -> ()  [unwired: 1 out]
        n64 = feedback #1() -> (w728:bool)  [unwired: 1 in]
        n65 = Not(x=w728) -> (.not. x?=w727:bool)
        n66 = feedback-in #1(w721) -> ()
        n67 = And(x=w727, y=w721) -> (x .and. y?=w723:bool)
        n68 = feedback #2() -> (w720:i32)  [unwired: 1 in]
        n69 = Select(t=w722, s=w723, f=w720) -> (s? t:f=w724:i32)
        n70 = feedback-in #2(w724) -> ()
        n71 = local read "Stop Button"() -> (w733:bool)
        n72 = Subtract(x=w722, y=w724) -> (x-y=w725:i32)
        n73 = Equal?(x=w725, y=2) -> (x = y?=w719:bool)
        n74 = case shown="True" w719 {
          frame False {
          }
          frame True {
            n75 = local write "Start Button"(FALSE ("Start Button")) -> ()
          }
        }
      }
      n76 = timed-loop {
        shift-right: [w121] -> _
        shift-left: TRUE -> [w133]
        shift-right: [w122] -> _
        shift-left: 0 -> [w118]
        shift-right: [w125] -> _
        shift-left: w88 -> [w131]
        tunnel: w73 -> [w117]
        timing: w77 -> [_]
        timing-out: [_] -> w76
        stop <- w138 stop-if-true
        # "Главный цикл"
        n77 = node-c288() -> (w116:errorcluster)  [unwired: 1 in]
        n78 = Tick Count (ms)() -> (millisecond timer value=w137:u32)
        n79 = Index Array(array=w131, index=w118) -> (element=w126:T23)
        n80 = Bundle By Name(cluster=w126, "Activ"=TRUE) -> (w127:T23)
        n81 = Replace Array Subset(array=w131, new element=w127, index=w118) -> (w132:T3)
        n82 = local write "Array 0"(w132) -> ()
        n83 = feedback #3() -> (w135:u32)  [unwired: 1 in]
        n84 = Select(t=w137, s=w133, f=w135) -> (s? t:f=w136:u32)
        n85 = feedback-in #3(w136) -> ()
        n86 = Unbundle By Name(w126) -> ("Skip"=w130:bool, "action"=w129:T2)
        n87 = call <vilib>:"Update VMX Data.vi"("error in (no error)"=w116) -> ("error out"=w115:errorcluster)  [unwired: 10 in]
        n88 = Subtract(x=w137, y=w136) -> (x-y=w134:u32)
        n89 = Select(t=Action_control."End" ("action"), s=w130, f=w129) -> (s? t:f=w123:T2)
        n90 = case shown="\"Gamepad\"" w123 {
          tunnel: w134 -> [w148 w159 _ w177 _ _ w283 w305 _ w334 _ _ _ _ w484 w544 _]
          tunnel: w133 -> [_ _ _ w169 _ w233 _ _ w318 w331 _ _ _ _ w463 w547 _]
          tunnel: w118 -> [_ _ _ _ _ _ _ _ _ _ _ w380 _ w410 _ _ _]
          tunnel: w131 -> [w151 w162 w166 w179 w195 w276 w287 w311 w319 w338 w372 w378 w409 w419 w459 w549 w575]
          tunnel: w126 -> [w149 w163 _ _ w194 _ w288 w310 _ w337 w368 w392 _ w420 w497 w548 _]
          tunnel: [w151 w162 w166 w179 w195 w276 w287 w311 w319 w338 w372 w378 w409 w411 w459 w549 w575] -> w125
          tunnel: [w144 w157 TRUE w171 w192 FALSE w279 w304 w318 w320 w365 TRUE TRUE TRUE w452 w524 TRUE] -> w121
          tunnel: [1 1.0 ("f") 1 1 1 1 1 1.0 ("f") 0 1 1.0 ("f") w379 1 0 1 1.0 ("f") 0] -> w120
          tunnel: w117 -> [_ _ _ _ _ w232 _ _ _ w333 _ _ _ _ w498 _ _]
          frame "Pause" {
            # "Пауза"
            n91 = Unbundle By Name(w149) -> ("X"=w146:dbl)  [unwired: 3 out]
            n92 = Divide(x=w148, y=u32 1000) -> (x/y=w145:dbl)
            n93 = Greater?(x=w145, y=w146) -> (0:w144:bool)
          }
          frame "Smooth pause" {
            n94 = Unbundle By Name(w163) -> ("X"=w158:dbl, "Y"=w155:dbl)
            n95 = Divide(x=w159, y=u32 1000) -> (x/y=w160:dbl)
            n96 = Greater?(x=w160, y=w158) -> (0:w157:bool)
            n97 = Bundle By Name(cluster=T7 {"M Left"=0.0, "M Right"=0.0, "M Back"=0.0} ("Motors"), "M Left"=w155, "M Right"=w155, "M Back"=w155) -> (w153:T7)
            n98 = local write "Motors"(w153) -> ()
            n99 = local write "Break"(FALSE ("Break")) -> ()
          }
          frame "Initialization" {
          }
          frame "Start", Default {
            w178 = T4 0 items=["Script 0", "Script 1", "Script 2", "Script 3", "Script 4", "Script 5", "Script 6", "Script 7", "Script 8", "Script 9", "Script 10", "Script 11", "Script 12", "Script 13", "Script 14", "Script 15", "Script 16", "Script 17", "Script 18", "Script 19", "Script 20", "Script 21", "Script 22", "Script 23", "Script 24", "Script 25", "Script 26", "Script 27"] ("Tab True")
            # "TRUE:  Зелёный светодиод горит - кнопка старт нажата"
            # "TRUE: Красный светодиод горит - ожидает нажатия кнопки старт"
            # "При ожидании нажатия кнопки \"Старт\" горит красный светодиод, зелёный погашен.\nПосле нажатия кнопки, оба светодиода загораются.\nSet 1: true -\nSet 2: true - \nSet 3: true -"
            # "Ожидание кнопки Старт"
            n100 = Divide(x=w177, y=u32 1000) -> (x/y=w175:dbl)
            n101 = case shown="True" w169 {
              frame False {
              }
              frame True {
                n102 = local read "Lift parameters"() -> (w182:T5)
                n103 = local write "Lift Reset"(TRUE ("Lift Reset")) -> ()
                n104 = Unbundle By Name(w182) -> ("Limit L"=w181:dbl)
                n105 = Increment(x=w181) -> (x+1=w180:dbl)
                n106 = local write "Lift Level"(w180) -> ()
              }
            }
            n107 = Greater Or Equal?(x=w175, y=5.0) -> (x >= y?=w172:bool)
            n108 = local write "Tab Script"(w178) -> ()
            n109 = local write "Break"(TRUE ("Break")) -> ()
            n110 = local read "Start Button"() -> (w173:bool)
            n111 = And(x=w173, y=w172) -> (x .and. y?=w171:bool)
            n112 = case shown="False" w172 {
              frame False {
                n113 = local write "Blink Red"(FALSE ("Blink Red")) -> ()
                n114 = local write "LED Red"(FALSE) -> ()
              }
              frame True {
                n115 = local write "Blink Red"(FALSE ("Blink Red")) -> ()
                n116 = local write "LED Red"(TRUE) -> ()
              }
            }
            n117 = case shown="False" w171 {
              frame False {
                n118 = local write "Blink Green"(FALSE ("Blink Red")) -> ()
                n119 = local write "LED Green"(FALSE) -> ()
              }
              frame True {
                n120 = local write "Blink Green"(FALSE ("Blink Red")) -> ()
                n121 = local write "LED Green"(TRUE) -> ()
              }
            }
            n122 = local write "Servo"(28.0 ("Servo")) -> ()
          }
          frame "Camera" {
            # "Команды для отладки и переноса файлов\n\nfdisk -l  - проверка активных устройств\nmount /dev/sda1 /media/usb - Монтирование флешки /dev/sda1 в директорию /media/usb\numount /dev/sda1 /media/usb - Размонтирование флешки /dev/sda1 из директории /media/usb\npython save.py test.png - запуск скрипта для сохранения изображения с камеры с названием файла test.png"
            # "Распознавание доски заказов и чтение результата"
            n123 = Unbundle By Name(w194) -> ("Set 1"=w193:bool)
            n124 = flat-sequence {
              tunnel: w193 -> [w197]
              tunnel: [TRUE] -> w192
              frame #0 {
                n125 = case shown="True" w197 {
                  frame False {
                  }
                  frame True {
                    # "Рабочая директория"
                    # "Запуск скрипта для распознавания доски заказов\n и чтение результата"
                    n126 = call <vilib>:"System Exec.vi"("working directory"=path "/home/pi", "command line"="python camera.py 1.png 2.png 3.png 4.png") -> ()  [unwired: 6 in, 4 out]
                  }
                }
              }
              frame #1 {
                n127 = call <vilib>:"System Exec.vi"("working directory"=path "/home/pi", "command line"="cat result.txt") -> ("standard output"=w200:string)  [unwired: 6 in, 3 out]
                n128 = local write "Camera result"(w200) -> ()
              }
              frame #2 {
                n129 = for {
                  N: 6 -> [_]
                  tunnel: [w216] -> w206 mode=indexing
                  i -> [w214]
                  n130 = Multiply(x=6, y=w214) -> (x*y=w215:i32)
                  n131 = for {
                    N: 6 -> [_]
                    tunnel: [w222] -> w216 mode=indexing
                    tunnel: w215 -> [w218]
                    i -> [w220]
                    n132 = local read "String to array"() -> (w221:dbl[])
                    n133 = Add(x=w218, y=w220) -> (x+y=w219:i32)
                    n134 = Index Array(array=w221, index=w219) -> (element=w222:dbl)
                  }
                }
                n135 = local read "String to array"() -> (w204:dbl[])
                n136 = local read "Camera result"() -> (w209:string)
                n137 = Index Array(array=w204, index="index") -> (element=→"element":dbl)
                n138 = Spreadsheet String To Array(delimiter (Tab)=";", format string="", spreadsheet string=w209, array type (2D Dbl)=dbl[] []) -> (array=w208:dbl[])
                n139 = local write "String to array"(w208) -> ()
                n140 = local write "Order Board"(w206) -> ()
              }
              frame #3 {
              }
            }
          }
          frame "Gamepad" {
            # "26.5"
            # "Движение"
            # "серво"
            # "Тест управления лифтом с геймпада"
            # "Работа с Gamepad"
            n141 = Unbundle By Name(w232) -> ("Gyroscope"=w231:refnum<class "IMU.lvclass">)
            n142 = call "Gyroscope.vi"("Reset YAW"=w233, "IMU in"=w231) -> ()  [unwired: 5 in, 5 out]
            n143 = local read "Joystick"() -> (w275:T10)
            n144 = Unbundle By Name(w275) -> ("X"=w246:bool, "B"=w257:bool, "X Right"=w226:i8, "Y Right"=w225:i8, "Back"=w230:bool, "0"=w235:bool, "180"=w234:bool)  [unwired: 9 out]
            "Y Right" <- w225
            "X Right" <- w226
            n145 = Negate(x=w226) -> (-x=w245:i8)
            n146 = Multiply(x=w245, y=-1) -> (x*y=w271:i32)
            n147 = feedback #4() -> (w242:dbl)  [unwired: 1 in]
            n148 = Add(x=0.01 ("t"), y=w242) -> (x+y=w243:dbl)
            n149 = Select(t=w243, s=w235, f=w242) -> (s? t:f=w239:dbl)
            n150 = Subtract(x=w239, y=0.01 ("t")) -> (x-y=w241:dbl)
            n151 = Select(t=w241, s=w234, f=w239) -> (s? t:f=w229:dbl)
            n152 = Divide(x=w245, y=2) -> (x/y=w258:dbl)
            n153 = Compound Arithmetic op=ADD(w225, w245) -> (w261:i8)
            n154 = Select(t=0.0, s=w230, f=w229) -> (s? t:f=w228:dbl)
            n155 = Compound Arithmetic op=ADD(w225, w271) -> (w265:i32)
            n156 = In Range and Coerce(upper limit=33.5, x=w228, lower limit=0.0) -> (coerced(x)=w236:dbl)  [unwired: 1 out]
            "coerced(x)" <- w236
            n157 = feedback-in #4(w236) -> ()
            n158 = In Range and Coerce(upper limit=50, x=w261, lower limit=-50) -> (coerced(x)=w260:i32)  [unwired: 1 out]
            n159 = In Range and Coerce(upper limit=50, x=w265, lower limit=-50) -> (coerced(x)=w264:i32)  [unwired: 1 out]
            n160 = In Range and Coerce(upper limit=50, x=w258, lower limit=-50) -> (coerced(x)=w259:dbl)  [unwired: 1 out]
            n161 = Bundle By Name(cluster=T7 {"M Left"=0.0, "M Right"=0.0, "M Back"=0.0} ("Motors"), "M Left"=w264, "M Right"=w260, "M Back"=w259) -> (w273:T7)
            n162 = local write "Lift Level"(w236) -> ()
            n163 = local write "Motors"(w273) -> ()
            n164 = feedback #5() -> (w248:dbl)  [unwired: 1 in]
            n165 = Add(x=1.0, y=w248) -> (x+y=w253:dbl)
            n166 = Select(t=w253, s=w246, f=w248) -> (s? t:f=w255:dbl)
            n167 = Subtract(x=w255, y=1.0) -> (x-y=w256:dbl)
            n168 = Select(t=w256, s=w257, f=w255) -> (s? t:f=w249:dbl)
            n169 = In Range and Coerce(upper limit=27.0, x=w249, lower limit=24.5) -> (coerced(x)=w247:dbl)  [unwired: 1 out]
            n170 = feedback-in #5(w247) -> ()
            n171 = local write "Servo"(w247) -> ()
            n172 = local write "Break"(FALSE ("Break")) -> ()
          }
          frame "OMS" {
            # "Серво"
            # "Лифт"
            n173 = Unbundle By Name(w288) -> ("X"=w286:dbl, "Y"=w285:dbl)  [unwired: 2 out]
            n174 = Divide(x=w283, y=1000.0) -> (x/y=w282:dbl)
            n175 = Greater?(x=w282, y=10.0) -> (0:w279:bool)
            n176 = case shown="1, Default" w285 {
              tunnel: w285 -> [_ w289]
              frame 0 {
              }
              frame 1, Default {
                n177 = local read "Lift parameters"() -> (w293:T5)
                n178 = Unbundle By Name(w293) -> ("Limit H"=w291:dbl, "Limit L"=w290:dbl)
                n179 = In Range and Coerce(upper limit=w291, x=w289, lower limit=w290) -> (coerced(x)=w292:dbl)  [unwired: 1 out]
                n180 = local write "Lift Level"(w292) -> ()
              }
            }
            n181 = case shown="2" w286 {
              frame 0, Default {
              }
              frame 1 {
                n182 = local read "ServoA"() -> (w295:dbl[])
                n183 = Index Array(array=w295, index=0) -> (element=w294:dbl)
                n184 = local write "Servo"(w294) -> ()
              }
              frame 2 {
                n185 = local read "ServoA"() -> (w298:dbl[])
                n186 = Index Array(array=w298, index=1) -> (element=w297:dbl)
                n187 = local write "Servo"(w297) -> ()
              }
              frame 3 {
                n188 = local read "ServoA"() -> (w301:dbl[])
                n189 = Index Array(array=w301, index=2) -> (element=w300:dbl)
                n190 = local write "Servo"(w300) -> ()
              }
            }
          }
          frame "Lift" {
            n191 = Unbundle(w310) -> ("X"=w309:dbl)  [unwired: 9 out]
            n192 = Divide(x=w305, y=1000.0) -> (x/y=w307:dbl)
            n193 = Greater?(x=w307, y=6.0) -> (0:w304:bool)
            n194 = case shown="4" w309 {
              frame 0, Default {
                n195 = local write "Lift Level"(0.0 ("Lift Level")) -> ()
              }
              frame 1 {
                n196 = local write "Lift Level"(3.0 ("Lift Level")) -> ()
              }
              frame 2 {
                n197 = local write "Lift Level"(17.0 ("Lift Level")) -> ()
              }
              frame 3 {
                n198 = local write "Lift Level"(32.0 ("Lift Level")) -> ()
              }
              frame 4 {
                n199 = local write "Lift Level"(7.0 ("Lift Level")) -> ()
              }
            }
          }
          frame "autonomus" {
          }
          frame "Rotation" {
            # "Вращение с гироскопом"
            n200 = Unbundle By Name(w333) -> ("Gyroscope"=w332:refnum<class "IMU.lvclass">)
            n201 = case shown="True" w331 {
              frame False {
              }
              frame True {
                # "Врубить моторы!"
                n202 = local write "Break"(FALSE ("Break")) -> ()
                n203 = local write "Block Rotate"(TRUE ("Block Rotate")) -> ()
              }
            }
            n204 = Unbundle By Name(w337) -> ("X"=w322:dbl)  [unwired: 3 out]
            n205 = Divide(x=w334, y=1000.0) -> (x/y=w325:dbl)
            n206 = call "Gyroscope.vi"("Reset YAW"=w331, "IMU in"=w332) -> ("YAW (degree)"=w326:dbl)  [unwired: 5 in, 4 out]
            "YAW (degree) 2" <- w326
            n207 = Absolute Value(x=w322) -> (abs(x)=w323:dbl)
            n208 = Greater?(x=w325, y=0.5) -> (0:w328:bool)
            n209 = Absolute Value(x=w326) -> (abs(x)=w321:dbl)
            n210 = In Range and Coerce(upper limit=w323, x=w321, lower limit=0.0) -> (In Range?=w324:bool)  [unwired: 1 out]
            n211 = case shown="True" w324 {
              tunnel: w322 -> [_ w351]
              tunnel: w321 -> [_ w340]
              frame False {
                n212 = local write "Break"(TRUE ("Break")) -> ()
              }
              frame True {
                n213 = Greater Or Equal To 0?(x=w351) -> (x >= 0?=w345:bool)
                n214 = Select(t=10.0, s=w345, f=-10.0) -> (s? t:f=w344:dbl)
                n215 = Select(t=40.0, s=w345, f=-40.0) -> (s? t:f=w348:dbl)
                n216 = In Range and Coerce(upper limit=83.0, x=w340, lower limit=60.0) -> (In Range?=w342:bool)  [unwired: 1 out]
                n217 = Not(x=w342) -> (.not. x?=w341:bool)
                n218 = Select(t=w348, s=w341, f=w344) -> (s? t:f=w343:dbl)
                "Waveform Chart 2" <- w343
                n219 = Negate(x=w343) -> (-x=w354:dbl)
                n220 = Bundle By Name(cluster=T7 {"M Left"=0.0, "M Right"=0.0, "M Back"=0.0} ("Motors"), "M Left"=w354, "M Right"=w343, "M Back"=w343) -> (w355:T7)
                n221 = local write "Motors"(w355) -> ()
              }
            }
            n222 = Not(x=w324) -> (.not. x?=w329:bool)
            n223 = And(x=w329, y=w328) -> (x .and. y?=w320:bool)
            n224 = case shown="True" w320 {
              frame False {
              }
              frame True {
                # "Вырубить моторы!"
                n225 = local write "Break"(TRUE ("Break")) -> ()
                n226 = local write "Block Rotate"(FALSE ("Block Rotate")) -> ()
              }
            }
          }
          frame "Rotation Correct" {
            n227 = Unbundle By Name(w368) -> ("X"=w363:dbl)
            n228 = local read "YAW (degree)"() -> (w364:dbl)
            n229 = call "Gyroscope Correct.vi"("Check"=w363, "YAW"=w364) -> ("Out motor"=w361:dbl, "Ok"=w362:bool)  [unwired: 1 in]
            n230 = case shown="True" w362 {
              tunnel: [FALSE ("Break") w374] -> w365
              frame False {
              }
              frame True {
                w374 = TRUE ("Break")
                n231 = local write "Break"(w374) -> ()
              }
            }
            n232 = Negate(x=w361) -> (-x=w369:dbl)
            n233 = Bundle By Name(cluster=T7 {"M Left"=0.0, "M Right"=0.0, "M Back"=0.0} ("Motors"), "M Left"=w369, "M Right"=w361, "M Back"=w361) -> (w370:T7)
            n234 = local write "Motors"(w370) -> ()
            n235 = local write "Break"(FALSE ("Break")) -> ()
          }
          frame "Go to" {
            n236 = Unbundle By Name(w392) -> ("X"=w384:dbl, "Y"=w391:dbl, "Z"=w387:dbl, "Div"=w377:i8, "Set 1"=w385:bool)  [unwired: 3 out]
            "Div" <- w377
            n237 = call "viayka.vi"("Num"=w377, "Array"=w378) -> ("Num Out"=w375:i32)  [unwired: 9 in]
            "Action" <- w375
            n238 = case shown="False" w385 {
              tunnel: w391 -> [w393 w394]
              tunnel: [w393 w394] -> w390
              frame False {
              }
              frame True {
              }
            }
            n239 = Subtract(x=w375, y=w380) -> (x-y=w381:dbl)
            "x-y" <- w381
            n240 = To Unsigned Byte Integer(number=w384) -> (unsigned 8bit integer=w383:u8)
            n241 = To Unsigned Byte Integer(number=w387) -> (unsigned 8bit integer=w386:u8)
            n242 = case shown="1" w383 {
              tunnel: [w401 w403] -> w382
              frame 0, Default {
                n243 = local read "Blink Green"() -> (w402:bool)
                n244 = Boolean To (0,1)(Boolean=w402) -> (0, 1=w401:i16)
              }
              frame 1 {
                n245 = local read "Blink Green"() -> (w404:bool)
                n246 = Boolean To (0,1)(Boolean=w404) -> (0, 1=w403:i16)
              }
            }
            n247 = case shown="1" w386 {
              tunnel: w390 -> [w396 w400]
              tunnel: [w395 w399] -> w388
              tunnel: w382 -> [w397 w398]
              frame 0, Default {
                n248 = Equal?(x=w397, y=w396) -> (x = y?=w395:bool)
              }
              frame 1 {
                n249 = Equal?(x=w398, y=w400) -> (x = y?=w399:bool)
              }
            }
            n250 = Select(t=w381, s=w388, f=1.0) -> (s? t:f=w379:dbl)
            "s? t:f" <- w379
          }
          frame "Empty script" {
            n251 = local read "String to array"() -> (w406:dbl[])
            n252 = Array Size(array=w406) -> (size(s)=→"size(s)":i32)
          }
          frame "Run scripts" {
            n253 = Unbundle By Name(w420) -> ("X"=w417:dbl)
            n254 = To Byte Integer(number=w417) -> (8bit integer=w414:i8)
            n255 = case shown="23" w414 {
              tunnel: ["Array Null" w422 w423 w424 w425 w426 w427 w428 w429 w430 w431 w432 w433 w434 w435 w436 w437 w438 w439 w440 w441 w442 w443 w444 w445 w446 w447 w448] -> w412
              frame 0, Default {
              }
              frame 1 {
                n256 = local read "Array 1"() -> (w422:T3)
              }
              frame 2 {
                n257 = local read "Array 2"() -> (w423:T3)
              }
              frame 3 {
                n258 = local read "Array 3"() -> (w424:T3)
              }
              frame 4 {
                n259 = local read "Array 4"() -> (w425:T3)
              }
              frame 5 {
                n260 = local read "Array 5"() -> (w426:T3)
              }
              frame 6 {
                n261 = local read "Array 6"() -> (w427:T3)
              }
              frame 7 {
                n262 = local read "Array 7"() -> (w428:T3)
              }
              frame 8 {
                n263 = local read "Array 8"() -> (w429:T3)
              }
              frame 9 {
                n264 = local read "Array 9"() -> (w430:T3)
              }
              frame 10 {
                n265 = local read "Array 10"() -> (w431:T3)
              }
              frame 11 {
                n266 = local read "Array 11"() -> (w432:T3)
              }
              frame 12 {
                n267 = local read "Array 12"() -> (w433:T3)
              }
              frame 13 {
                n268 = local read "Array 13"() -> (w434:T3)
              }
              frame 14 {
                n269 = local read "Array 14"() -> (w435:T3)
              }
              frame 15 {
                n270 = local read "Array 15"() -> (w436:T3)
              }
              frame 16 {
                n271 = local read "Array 16"() -> (w437:T3)
              }
              frame 17 {
                n272 = local read "Array 17"() -> (w438:T3)
              }
              frame 18 {
                n273 = local read "Array 18"() -> (w439:T3)
              }
              frame 19 {
                n274 = local read "Array 19"() -> (w440:T3)
              }
              frame 20 {
                n275 = local read "Array 20"() -> (w441:T3)
              }
              frame 21 {
                n276 = local read "Array 21"() -> (w442:T3)
              }
              frame 22 {
                n277 = local read "Array 22"() -> (w443:T3)
              }
              frame 23 {
                n278 = local read "Array 23"() -> (w444:T3)
              }
              frame 24 {
                n279 = local read "Array 24"() -> (w445:T3)
              }
              frame 25 {
                n280 = local read "Array 25"() -> (w446:T3)
              }
              frame 26 {
                n281 = local read "Array 26"() -> (w447:T3)
              }
              frame 27 {
                n282 = local read "Array 27"() -> (w448:T3)
              }
            }
            n283 = Delete From Array(array=w419, length=1 ("index"), index=w410) -> (array with subset deleted=w413:T3)  [unwired: 1 out]
            n284 = Insert Into Array(array=w413, index=w410, new element=w412) -> (w411:T3)
          }
          frame "Move" {
            w478 = 0.5 ("upper limit")
            n285 = Unbundle By Name(w498) -> ("TitanENC"=w496:T21)
            n286 = Unbundle By Name(w497) -> ("X"=w453:dbl, "Y"=w449:dbl)  [unwired: 1 out]
            n287 = local read "Motors Renum"() -> (w495:cluster{"Num":i32, "Directly":bool, "KM":dbl}[])
            n288 = Divide(x=w484, y=u32 1000) -> (x/y=w481:dbl)
            n289 = case shown="True" w463 {
              frame False {
              }
              frame True {
                n290 = local write "Break"(FALSE ("Break")) -> ()
              }
            }
            n291 = In Range and Coerce(upper limit=w478, x=w481, lower limit=0.0) -> (coerced(x)=w479:dbl)  [unwired: 1 out]
            n292 = call "Encoders Read.vi"("Motors Renum"=w495, "Start"=w463, "TitanENC in"=w496) -> ("ENC True"=w458:T6)  [unwired: 3 in, 5 out]
            n293 = Greater?(x=w481, y=0.5) -> (0:w460:bool)
            n294 = Unbundle By Name(w458) -> ("ENC Left"=w494:i32, "ENC Right"=w493:i32, "ENC Back"=w492:i32)
            n295 = Divide(x=w479, y=w478) -> (x/y=w476:dbl)
            n296 = Multiply(x=50.0, y=w476) -> (x*y=w474:dbl)
            n297 = Bundle By Name(cluster=T7 {"M Left"=0.0, "M Right"=0.0, "M Back"=0.0} ("Motors"), "M Left"=w494, "M Right"=w493, "M Back"=w492) -> (w490:T7)
            n298 = local read "Factor"() -> (w489:cluster{"Kx":dbl, "Kz":dbl, "Ky":dbl})
            n299 = Absolute Value(x=w453) -> (abs(x)=w486:dbl)
            n300 = call "Enc to XY.vi"("Factor"=w489, "Encoders"=w490) -> ("Distance"=w488:cluster{"X":dbl, "Y":dbl})  [unwired: 8 in, 1 out]
            n301 = Subtract(x=w486, y=1.0) -> (x-y=w467:dbl)
            n302 = Absolute Value(x=w488) -> (abs(x)=w487:cluster{"X":dbl, "Y":dbl})
            n303 = Unbundle By Name(w487) -> ("X"=→"X":dbl, "Y"=w466:dbl)
            "Y" <- w466
            n304 = Subtract(x=w467, y=w466) -> (x-y=w470:dbl)
            n305 = Multiply(x=w470, y=8.0) -> (x*y=w472:dbl)
            n306 = In Range and Coerce(upper limit=w472, x=w472, lower limit=0.0) -> (coerced(x)=w473:dbl)  [unwired: 1 out]
            n307 = Less?(x=w473, y=w474) -> (x < y?=w475:bool)
            n308 = Select(t=w473, s=w475, f=w474) -> (s? t:f=w457:dbl)
            "move ind" <- w457
            n309 = In Range and Coerce(upper limit=w467, x=w466, lower limit=0.0) -> (In Range?=w464:bool)  [unwired: 1 out]
            n310 = case shown="True" w464 {
              tunnel: w453 -> [_ w515]
              tunnel: w457 -> [_ w516]
              frame False {
                w507 = 0.0 ("M Left")
                n311 = Bundle By Name(cluster=T7 {"M Left"=0.0, "M Right"=0.0, "M Back"=0.0} ("Motors"), "M Left"=w507, "M Right"=w507, "M Back"=w507) -> (w509:T7)
                n312 = local write "Motors"(w509) -> ()
              }
              frame True {
                n313 = Negate(x=w516) -> (-x=w514:dbl)
                n314 = Greater Than 0?(x=w515) -> (x > 0?=w517:bool)
                n315 = Select(t=w516, s=w517, f=w514) -> (s? t:f=w511:dbl)
                n316 = Bundle By Name(cluster=T7 {"M Left"=0.0, "M Right"=0.0, "M Back"=0.0} ("Motors"), "M Left"=w511, "M Right"=w511, "M Back"=0.0) -> (w513:T7)
                n317 = local write "Motors"(w513) -> ()
              }
            }
            n318 = Not(x=w464) -> (.not. x?=w462:bool)
            n319 = Not(x=w463) -> (.not. x?=w461:bool)
            n320 = local read "IR median"() -> (w455:dbl)
            n321 = Less Or Equal?(x=w455, y=w449) -> (x <= y?=w454:bool)
            n322 = case shown="True" w454 {
              tunnel: [FALSE ("wall stop") TRUE ("wall stop")] -> w451
              frame False {
                n323 = local write "wall stop"(FALSE ("wall stop")) -> ()
                n324 = local write "Break"(FALSE ("Break")) -> ()
              }
              frame True {
                n325 = local write "wall stop"(TRUE ("wall stop")) -> ()
                n326 = local write "Break"(TRUE ("Break")) -> ()
              }
            }
            n327 = Compound Arithmetic op=AND(w462, w461, w460) -> (w450:bool)
            n328 = case shown="True" w450 {
              frame False {
              }
              frame True {
                n329 = local write "Break"(TRUE ("Break")) -> ()
              }
            }
            n330 = Or(x=w451, y=w450) -> (x .or. y?=w452:bool)
          }
          frame "Move GPS" {
            w541 = 0.5 ("upper limit")
            n331 = Unbundle By Name(w548) -> ("X"=w518:dbl)
            n332 = Add(x=w544, y=1000.0) -> (x+y=w523:dbl)
            n333 = Greater Than 0?(x=w518) -> (x > 0?=w546:bool)
            n334 = case shown="True" w547 {
              frame False {
              }
              frame True {
                n335 = local write "Block Rotate"(TRUE ("Block Rotate")) -> ()
                n336 = local write "Break"(FALSE ("Break")) -> ()
              }
            }
            n337 = Greater?(x=w523, y=0.5) -> (0:w522:bool)
            n338 = local read "YAW (degree)"() -> (w529:dbl)
            n339 = In Range and Coerce(upper limit=w541, x=w523, lower limit=0.0) -> (coerced(x)=w542:dbl)  [unwired: 1 out]
            n340 = Divide(x=w542, y=w541) -> (x/y=w540:dbl)
            n341 = Multiply(x=30.0, y=w540) -> (x*y=w536:dbl)
            n342 = Round Toward +Infinity(x=w518) -> (ceil(x): smallest int >= x=w531:dbl)
            n343 = Round Toward +Infinity(x=w529) -> (ceil(x): smallest int >= x=w526:dbl)
            n344 = Subtract(x=w531, y=3.5) -> (x-y=w527:dbl)
            n345 = Subtract(x=w527, y=w526) -> (x-y=w532:dbl)
            n346 = In Range and Coerce(upper limit=w532, x=w532, lower limit=0.0) -> (coerced(x)=w534:dbl)  [unwired: 1 out]
            n347 = Less?(x=w534, y=w536) -> (x < y?=w537:bool)
            n348 = Select(t=w534, s=w537, f=w536) -> (s? t:f=w535:dbl)
            n349 = case shown="False" w546 {
              tunnel: w535 -> [w565 w567]
              tunnel: [w565 w566] -> w525
              frame False {
              }
              frame True {
                n350 = Negate(x=w567) -> (-x=w566:dbl)
              }
            }
            n351 = In Range and Coerce(upper limit=w527, x=w526, lower limit=0.0) -> (In Range?=w520:bool)  [unwired: 1 out]
            n352 = Not(x=w520) -> (.not. x?=w519:bool)
            n353 = And(x=w519, y=w522) -> (x .and. y?=w524:bool)
            n354 = case shown="False" w520 {
              tunnel: w525 -> [_ w561]
              frame False {
              }
              frame True {
                n355 = Negate(x=w561) -> (-x=w562:dbl)
                n356 = Bundle By Name(cluster=T7 {"M Left"=0.0, "M Right"=0.0, "M Back"=0.0} ("Motors"), "M Left"=w562, "M Right"=w561, "M Back"=w561) -> (w563:T7)
                n357 = local write "Motors"(w563) -> ()
              }
            }
            n358 = case shown="True" w524 {
              tunnel: w518 -> [_ w555]
              frame False {
              }
              frame True {
                n359 = local read "GPS"() -> (w560:cluster{"X":dbl, "Y":dbl, "Angle ":i16})
                n360 = feedback #6(0.0) -> (w556:dbl)
                n361 = Add(x=w556, y=w555) -> (x+y=w557:dbl)
                n362 = feedback-in #6(w557) -> ()
                n363 = Unbundle By Name(w560) -> ("X"=w554:dbl, "Y"=w553:dbl)
                n364 = local write "Block Rotate"(FALSE) -> ()
                n365 = local write "Break"(TRUE) -> ()
                n366 = Bundle By Name(cluster=cluster{"X":dbl, "Y":dbl, "Angle ":i16} {"X"=0.0, "Y"=0.0, "Angle "=0} ("GPS"), "Angle"=w557, "X"=w554, "Y"=w553) -> (w558:cluster{"X":dbl, "Y":dbl, "Angle ":i16})
                n367 = local write "GPS"(w558) -> ()
              }
            }
          }
          frame "End" {
            w574 = FALSE ("LED Green")
            w573 = TRUE ("Break")
            # "Гашение всех светодидов и переход на завершение программы"
            # "Завершениние работы"
            n368 = local write "LED Green"(w574) -> ()
            n369 = local write "Break"(w573) -> ()
            n370 = local write "Stop Button"(w573) -> ()
            n371 = local write "LED Red"(w574) -> ()
            n372 = local write "Break"(TRUE ("Break")) -> ()
          }
        }
        n373 = Add(x=w120, y=w118) -> (x+y=w119:dbl)
        n374 = local read "Stop Button"() -> (w138:bool)
        n375 = node-c288(w115) -> ()  [unwired: 1 out]
        n376 = Select(t=w119, s=w121, f=w118) -> (s? t:f=w122:dbl)
      }
      n377 = node-c288() -> (w94:T11)  [unwired: 2 in]
      n378 = node-c288(w100) -> ()  [unwired: 1 out]
      n379 = node-c288(w78) -> ()  [unwired: 1 out]
      n380 = timed-loop {
        timing: w94 -> [_]
        timing-out: [_] -> w93
        tunnel: w73 -> [w706]
        tunnel: w81 -> [w703]
        stop <- w707 stop-if-true
        # "Управление сервомоторами"
        n381 = node-c288() -> (w709:errorcluster)  [unwired: 1 in]
        n382 = Unbundle By Name(w706) -> ("Servo"=w705:refnum<class "PWM.lvclass">)
        n383 = call <vilib>:"Update VMX Data.vi"("error in (no error)"=w709) -> ("error out"=w708:errorcluster)  [unwired: 10 in]
        n384 = local read "Stop Button"() -> (w707:bool)
        n385 = node-c288(w708) -> ()  [unwired: 1 out]
        n386 = call "Servo.vi"("error in (no error)"=w703, "Servo"="Servo", "PWM in"=w705) -> ()  [unwired: 6 in, 3 out]
      }
      n387 = node-c288() -> (w92:T11)  [unwired: 4 in]
      n388 = node-c288() -> (w75:T11)  [unwired: 4 in]
      n389 = timed-loop {
        timing: w92 -> [_]
        timing-out: [_] -> w91
        tunnel: w73 -> [w676]
        i -> [w683]
        stop <- w695 stop-if-true
        # "Управление светодиодами"
        n390 = node-c288() -> (w694:errorcluster)  [unwired: 1 in]
        n391 = local read "Blink Green"() -> (w686:bool)
        n392 = Unbundle By Name(w676) -> ("LEDs"=w692:T17, "Analog"=w675:T18)
        n393 = local read "LED Green"() -> (w688:bool)
        n394 = local read "Blink Red"() -> (w687:bool)
        n395 = Divide(x=w683, y=50) -> (x/y=w681:dbl)
        n396 = local read "LED Red"() -> (w689:bool)
        n397 = call "Analog.vi"("Analog In in"=w675) -> ("Volage"=→"Volage" →"Waveform Chart":dbl)  [unwired: 8 in, 2 out]
        n398 = To Long Integer(number=w681) -> (32bit integer=w680:i32)
        n399 = Quotient & Remainder(x=w680, y=2) -> (x-y*floor(x/y)=w678:i32)  [unwired: 1 out]
        n400 = call <vilib>:"Update VMX Data.vi"("error in (no error)"=w694) -> ("error out"=w693:errorcluster)  [unwired: 10 in]
        n401 = Equal To 0?(x=w678) -> (x = 0?=w677:bool)
        n402 = Not And(1:w677, 2:w687) -> (0:w685:bool)
        n403 = Not And(1:w677, 2:w686) -> (0:w684:bool)
        n404 = local read "Stop Button"() -> (w695:bool)
        n405 = And(x=w689, y=w685) -> (x .and. y?=w691:bool)
        n406 = And(x=w688, y=w684) -> (x .and. y?=w690:bool)
        n407 = node-c288(w693) -> ()  [unwired: 1 out]
        n408 = call "LED 2V2.vi"("Digital IO in"=w692, "LED Red"=w691, "LED Green"=w690) -> ()  [unwired: 11 in, 2 out]
      }
      n409 = timed-loop {
        timing: w75 -> [_]
        timing-out: [_] -> w74
        stop <- w107 stop-if-true
        # "GPS"
        # "GPS"
        n410 = node-c288() -> (w106:errorcluster)  [unwired: 1 in]
        n411 = local read "GPS"() -> (w103:cluster{"X":dbl, "Y":dbl, "Angle ":i16})
        n412 = call "GPS.vi"("GPS In"=w103, "Y"=0.0) -> ("GPS Out"=w102:cluster{"X":dbl, "Y":dbl, "Angle ":i16})
        n413 = call <vilib>:"Update VMX Data.vi"("error in (no error)"=w106) -> ("error out"=w105:errorcluster)  [unwired: 10 in]
        n414 = local write "GPS True"(w102) -> ()
        n415 = local read "Stop Button"() -> (w107:bool)
        n416 = node-c288(w105) -> ()  [unwired: 1 out]
      }
      n417 = node-c288(w93) -> ()  [unwired: 1 out]
      n418 = node-c288(w91) -> ()  [unwired: 1 out]
      n419 = node-c288() -> (w87:T11)  [unwired: 2 in]
      n420 = timed-loop {
        timing: w87 -> [_]
        timing-out: [_] -> w86
        tunnel: w73 -> [w664]
        stop <- w658 stop-if-true
        w659 = FALSE
        # "Управление лифтом"
        n421 = node-c288() -> (w666:errorcluster)  [unwired: 1 in]
        n422 = local read "Lift Level"() -> (w662:dbl)
        n423 = local read "ENC"() -> (w661:T6)
        n424 = local read "Lift parameters"() -> (w660:T5)
        n425 = Unbundle By Name(w664) -> ("Switch"=w663:T15)
        n426 = local read "Lift Reset"() -> (w653:bool)
        n427 = call <vilib>:"Update VMX Data.vi"("error in (no error)"=w666) -> ("error out"=w665:errorcluster)  [unwired: 10 in]
        n428 = call "Lift.vi"("Set H"=w659, "Set L"=w659, "Reset"=w653, "Lift parameters"=w660, "ENC"=w661, "Lift Level"=w662, "HG_LIB in"=w663) -> ("Reset Out"=w654:bool, "Lift in  Range"=w655:bool, "Lift True"=w656:dbl, "Lift Motor"=w657:dbl)  [unwired: 1 in]
        n429 = local read "Stop Button"() -> (w658:bool)
        n430 = local write "Lift Reset"(w654) -> ()
        n431 = local write "M Lift"(w657) -> ()
        n432 = local write "Lift in  Range"(w655) -> ()
        n433 = local write "Lift"(w656) -> ()
        n434 = node-c288(w665) -> ()  [unwired: 1 out]
      }
      n435 = node-c288(w74) -> ()  [unwired: 1 out]
      n436 = node-c288() -> (w85:T11)  [unwired: 2 in]
      n437 = timed-loop {
        timing: w85 -> [_]
        timing-out: [_] -> w84
        tunnel: w73 -> [w637]
        tunnel: w81 -> [w629]
        stop <- w643 stop-if-true
        # "Энкодеры"
        n438 = node-c288() -> (w645:errorcluster)  [unwired: 1 in]
        n439 = local read "Reset Enc"() -> (w628:bool)
        n440 = local read "PID gains"() -> (w627:T8)
        n441 = First Call?() -> (First Call?: T/F=w640:bool)
        n442 = local read "Motors Renum"() -> (w633:cluster{"Num":i32, "Directly":bool, "KM":dbl}[])
        n443 = Unbundle By Name(w637) -> ("TitanENC"=w642:T21)
        n444 = Unbundle By Name(w637) -> ("DC Motors"=w636:refnum<class "CAN.lvclass">)
        n445 = Or(x=w640, y=w628) -> (x .or. y?=w641:bool)
        n446 = call <vilib>:"Update VMX Data.vi"("error in (no error)"=w645) -> ("error out"=w644:errorcluster)  [unwired: 10 in]
        n447 = call "Encoders.vi"("Motors Renum"=w633, "error in (no error)"=w629, "Reset Enc"=w641, "Start"=w641, "TitanENC in"=w642) -> ("RPM"=w639:T9, "ENC True"=→"ENC True":T6, "ENC"=w634:T6)  [unwired: 1 in, 3 out]
        "RPM" <- w639
        n448 = local read "Motors"() -> (w631:T7)
        n449 = local read "M Lift"() -> (w632:dbl)
        n450 = local read "Stop Button"() -> (w643:bool)
        n451 = local read "Break"() -> (w626:bool)
        n452 = call "Speed PID 3 motors.vi"("dt (s)"=0.02, "M Lift"=w632, "error in (no error)"=w629, "PID gains"=w627, "Motors Real"=w639, "Motors"=w631) -> ("Motors Out"=w638:dbl[])  [unwired: 4 in, 1 out]
        n453 = local write "ENC"(w634) -> ()
        n454 = node-c288(w644) -> ()  [unwired: 1 out]
        n455 = call "DCMotors_All.vi"("Stop"=w626, "error in"=w629, "Motors Renum"=w633, "Input"=w638, "CAN in"=w636) -> ()  [unwired: 5 in, 2 out]
      }
      n456 = node-c288(w86) -> ()  [unwired: 1 out]
      n457 = node-c288() -> (w83:T11)  [unwired: 2 in]
      n458 = timed-loop {
        timing: w83 -> [_]
        timing-out: [_] -> w82
        tunnel: w73 -> [w609]
        stop <- w617 stop-if-true
        # "Гироскоп"
        n459 = node-c288() -> (w616:errorcluster)  [unwired: 1 in]
        n460 = local read "Block Rotate"() -> (w605:bool)
        n461 = Unbundle By Name(w609) -> ("Gyroscope"=w607:refnum<class "IMU.lvclass">)
        n462 = local read "ENC"() -> (w614:T6)
        n463 = Unbundle By Name(w614) -> ("ENC Left"=w612:i32, "ENC Right"=w611:i32, "ENC Back"=w610:i32)
        n464 = local read "Set GPS"() -> (w606:cluster{"Set":bool, "X":dbl, "Y":dbl, "Z":dbl})
        n465 = local read "Factor"() -> (w599:cluster{"Kx":dbl, "Kz":dbl, "Ky":dbl})
        n466 = local read "GPS"() -> (w600:cluster{"X":dbl, "Y":dbl, "Angle ":i16})
        n467 = Bundle By Name(cluster=T14 {"Enc Left"=0, "Enc Right"=0, "Enc Back"=0} ("Encoders"), "Enc Left"=w612, "Enc Right"=w611, "Enc Back"=w610) -> (w608:T14)
        n468 = call <vilib>:"Update VMX Data.vi"("error in (no error)"=w616) -> ("error out"=w615:errorcluster)  [unwired: 10 in]
        n469 = call "GPS Smart.vi"("Factor"=w599, "GPS"=w600, "Block Rotate"=w605, "Set GPS"=w606, "IMU in"=w607, "Encoders"=w608) -> ("Ok"=w603:bool, "Set GPS Out"=w601:cluster{"Set":bool, "X":dbl, "Y":dbl, "Z":dbl}, "GPS True Out"=w604:cluster{"X":dbl, "Y":dbl, "Z":dbl})  [unwired: 3 in]
        n470 = local write "GPS True"(w604) -> ()
        n471 = local read "Stop Button"() -> (w617:bool)
        n472 = feedback-in #7(w603) -> ()
        n473 = feedback #7() -> (w602:bool)  [unwired: 1 in]
        n474 = case shown="True" w602 {
          tunnel: w601 -> [_ w618]
          frame False {
          }
          frame True {
            n475 = local write "Set GPS"(w618) -> ()
          }
        }
        n476 = node-c288(w615) -> ()  [unwired: 1 out]
      }
      n477 = node-c288(w84) -> ()  [unwired: 1 out]
      n478 = node-c288(w82) -> ()  [unwired: 1 out]
      n479 = node-c288(w76) -> ()  [unwired: 1 out]
    }
    frame #2 {
      # "Close(Stop)"
      n480 = for {
        N: 5 -> [_]
        tunnel: w770 -> [w774]
        n481 = Unbundle By Name(w774) -> ("DC Motors"=w776:refnum<class "CAN.lvclass">)
        n482 = local read "Motors Renum"() -> (w777:cluster{"Num":i32, "Directly":bool, "KM":dbl}[])
        n483 = local read "Break"() -> (w778:bool)
        n484 = call "DCMotors_All.vi"("Stop"=w778, "Motors Renum"=w777, "Input"=dbl[] [0.0, 0.0, -0.01, 0.0], "CAN in"=w776) -> ()  [unwired: 6 in, 2 out]
      }
    }
    frame #3 {
      # "Сетевой адресс"
      # "Отключение портов"
      # "Отключение порта"
      # "End"
      n485 = Unbundle By Name(w803) -> ("Ir Sensor.Ir Sensor L"=w802:refnum<class "Analog In.lvclass">, "Ir Sensor.Ir Sensor R"=w801:refnum<class "Analog In.lvclass">, "Ultrasonic.Puls L"=w800:refnum<class "Pulse.lvclass">, "Ultrasonic.Eсho L"=w799:refnum<class "ISQ.lvclass">, "Ultrasonic.Puls R"=w798:refnum<class "Pulse.lvclass">, "Ultrasonic.Eсho R"=w787:refnum<class "ISQ.lvclass">, "Line Sensor"=w797:refnum<class "IIC.lvclass">, "DC Motors"=w796:refnum<class "CAN.lvclass">, "TitanENC.TitanENC 0"=w786:refnum<class "TitanENC.lvclass">, "TitanENC.TitanENC 1"=w795:refnum<class "TitanENC.lvclass">, "TitanENC.TitanENC 2"=w794:refnum<class "TitanENC.lvclass">, "TitanENC.TitanENC 3"=w785:refnum<class "TitanENC.lvclass">, "Switch.Limit H"=w793:refnum<class "Digital Input and Output.lvclass">, "Switch.Limit L"=w792:refnum<class "Digital Input and Output.lvclass">, "Buttons.Button Start"=w784:refnum<class "Digital Input and Output.lvclass">, "Buttons.Button Stop"=w791:refnum<class "Digital Input and Output.lvclass">, "LEDs.LED Red"=w790:refnum<class "Digital Input and Output.lvclass">, "LEDs.LED Green"=w783:refnum<class "Digital Input and Output.lvclass">, "Servo"=w779:refnum<class "PWM.lvclass">, "Analog.Analog"=w789:refnum<class "Analog In.lvclass">, "Analog.Voltage"=w782:refnum<class "Analog In.lvclass">, "Gyroscope"=w788:refnum<class "IMU.lvclass">)
      n486 = UDP Close(connection ID=w781, 8:w780) -> ()  [unwired: 2 out]
      n487 = call <vilib>:"Delete ID.vi"("HG_LIB in"=w802) -> ()  [unwired: 9 in, 2 out]
      n488 = call <vilib>:"Delete ID.vi"("HG_LIB in"=w799) -> ()  [unwired: 9 in, 2 out]
      n489 = call <vilib>:"Delete ID.vi"("HG_LIB in"=w797) -> ()  [unwired: 9 in, 2 out]
      n490 = call <vilib>:"Delete ID.vi"("HG_LIB in"=w795) -> ()  [unwired: 9 in, 2 out]
      n491 = call <vilib>:"Delete ID.vi"("HG_LIB in"=w793) -> ()  [unwired: 9 in, 2 out]
      n492 = call <vilib>:"Delete ID.vi"("HG_LIB in"=w791) -> ()  [unwired: 9 in, 2 out]
      n493 = call <vilib>:"Delete ID.vi"("HG_LIB in"=w788) -> ()  [unwired: 9 in, 2 out]
      n494 = call <vilib>:"Delete ID.vi"("HG_LIB in"=w779) -> ()  [unwired: 9 in, 2 out]
      n495 = call <vilib>:"Delete ID.vi"("HG_LIB in"=w800) -> ()  [unwired: 9 in, 2 out]
      n496 = call <vilib>:"Delete ID.vi"("HG_LIB in"=w787) -> ()  [unwired: 9 in, 2 out]
      n497 = call <vilib>:"Delete ID.vi"("HG_LIB in"=w786) -> ()  [unwired: 9 in, 2 out]
      n498 = call <vilib>:"Delete ID.vi"("HG_LIB in"=w785) -> ()  [unwired: 9 in, 2 out]
      n499 = call <vilib>:"Delete ID.vi"("HG_LIB in"=w784) -> ()  [unwired: 9 in, 2 out]
      n500 = call <vilib>:"Delete ID.vi"("HG_LIB in"=w783) -> ()  [unwired: 9 in, 2 out]
      n501 = call <vilib>:"Delete ID.vi"("HG_LIB in"=w782) -> ()  [unwired: 9 in, 2 out]
      n502 = call <vilib>:"Delete ID.vi"("HG_LIB in"=w801) -> ()  [unwired: 9 in, 2 out]
      n503 = call <vilib>:"Delete ID.vi"("HG_LIB in"=w798) -> ()  [unwired: 9 in, 2 out]
      n504 = call <vilib>:"Delete ID.vi"("HG_LIB in"=w796) -> ()  [unwired: 9 in, 2 out]
      n505 = call <vilib>:"Delete ID.vi"("HG_LIB in"=w794) -> ()  [unwired: 9 in, 2 out]
      n506 = call <vilib>:"Delete ID.vi"("HG_LIB in"=w792) -> ()  [unwired: 9 in, 2 out]
      n507 = call <vilib>:"Delete ID.vi"("HG_LIB in"=w790) -> ()  [unwired: 9 in, 2 out]
      n508 = call <vilib>:"Delete ID.vi"("HG_LIB in"=w789) -> ()  [unwired: 9 in, 2 out]
    }
  }
